vi "Config Info Get.vi"(8 "错误输入":errorcluster, 11 "Config Info":T8) -> (0 "错误输出":errorcluster, 1 "PLC Comms":T1={"PLC boolean read Tags"={"AT glass position"={"Tag Name"="S060.PXI.Signals.PlltData.SN", "Network Path"="172.15.51.1,1,0", "use opc"=FALSE, "DataSocket Reference"={"CWDSLib._DCWDataSocket"=refnum, "CWDSLib._DCWData"=refnum, "OnDataUpdated"=0, "OnStatusUpdated"=0}}, "AT shade position"={"Tag Name"="S060.PXI.Signals.PlltData.SN", "Network Path"="172.15.51.1,1,0", "use opc"=FALSE, "DataSocket Reference"={"CWDSLib._DCWDataSocket"=refnum, "CWDSLib._DCWData"=refnum, "OnDataUpdated"=0, "OnStatusUpdated"=0}}, "AT in glass wand lower pos"={"Tag Name"="S060.PXI.Signals.PlltData.SN", "Network Path"="172.15.51.1,1,0", "use opc"=FALSE, "DataSocket Reference"={"CWDSLib._DCWDataSocket"=refnum, "CWDSLib._DCWData"=refnum, "OnDataUpdated"=0, "OnStatusUpdated"=0}}, "AT in glass wand up pos"={"Tag Name"="S060.PXI.Signals.PlltData.SN", "Network Path"="172.15.51.1,1,0", "use opc"=FALSE, "DataSocket Reference"={"CWDSLib._DCWDataSocket"=refnum, "CWDSLib._DCWData"=refnum, "OnDataUpdated"=0, "OnStatusUpdated"=0}}, "AT in sunshad wand lower pos"={"Tag Name"="S060.PXI.Signals.PlltData.SN", "Network Path"="172.15.51.1,1,0", "use opc"=FALSE, "DataSocket Reference"={"CWDSLib._DCWDataSocket"=refnum, "CWDSLib._DCWData"=refnum, "OnDataUpdated"=0, "OnStatusUpdated"=0}}, "AT in sunshad wand up pos"={"Tag Name"="S060.PXI.Signals.PlltData.SN", "Network Path"="172.15.51.1,1,0", "use opc"=FALSE, "DataSocket Reference"={"CWDSLib._DCWDataSocket"=refnum, "CWDSLib._DCWData"=refnum, "OnDataUpdated"=0, "OnStatusUpdated"=0}}, "AT in wand home pos"={"Tag Name"="S060.PXI.Signals.PlltData.SN", "Network Path"="172.15.51.1,1,0", "use opc"=FALSE, "DataSocket Reference"={"CWDSLib._DCWDataSocket"=refnum, "CWDSLib._DCWData"=refnum, "OnDataUpdated"=0, "OnStatusUpdated"=0}}, "LVDT's Extended"={"Tag Name"="S060.PXI.Signals.PlltData.SN", "Network Path"="172.15.51.1,1,0", "use opc"=FALSE, "DataSocket Reference"={"CWDSLib._DCWDataSocket"=refnum, "CWDSLib._DCWData"=refnum, "OnDataUpdated"=0, "OnStatusUpdated"=0}}, "bolt check 1"={"Tag Name"="S060.PXI.Signals.PlltData.SN", "Network Path"="172.15.51.1,1,0", "use opc"=FALSE, "DataSocket Reference"={"CWDSLib._DCWDataSocket"=refnum, "CWDSLib._DCWData"=refnum, "OnDataUpdated"=0, "OnStatusUpdated"=0}}, "bolt check 2"={"Tag Name"="S060.PXI.Signals.PlltData.SN", "Network Path"="172.15.51.1,1,0", "use opc"=FALSE, "DataSocket Reference"={"CWDSLib._DCWDataSocket"=refnum, "CWDSLib._DCWData"=refnum, "OnDataUpdated"=0, "OnStatusUpdated"=0}}, "bolt check 3"={"Tag Name"="S060.PXI.Signals.PlltData.SN", "Network Path"="172.15.51.1,1,0", "use opc"=FALSE, "DataSocket Reference"={"CWDSLib._DCWDataSocket"=refnum, "CWDSLib._DCWData"=refnum, "OnDataUpdated"=0, "OnStatusUpdated"=0}}, "bolt check 4"={"Tag Name"="S060.PXI.Signals.PlltData.SN", "Network Path"="172.15.51.1,1,0", "use opc"=FALSE, "DataSocket Reference"={"CWDSLib._DCWDataSocket"=refnum, "CWDSLib._DCWData"=refnum, "OnDataUpdated"=0, "OnStatusUpdated"=0}}, "bolt check 5"={"Tag Name"="S060.PXI.Signals.PlltData.SN", "Network Path"="172.15.51.1,1,0", "use opc"=FALSE, "DataSocket Reference"={"CWDSLib._DCWDataSocket"=refnum, "CWDSLib._DCWData"=refnum, "OnDataUpdated"=0, "OnStatusUpdated"=0}}, "bolt check 6"={"Tag Name"="S060.PXI.Signals.PlltData.SN", "Network Path"="172.15.51.1,1,0", "use opc"=FALSE, "DataSocket Reference"={"CWDSLib._DCWDataSocket"=refnum, "CWDSLib._DCWData"=refnum, "OnDataUpdated"=0, "OnStatusUpdated"=0}}, "bolt check 7"={"Tag Name"="S060.PXI.Signals.PlltData.SN", "Network Path"="172.15.51.1,1,0", "use opc"=FALSE, "DataSocket Reference"={"CWDSLib._DCWDataSocket"=refnum, "CWDSLib._DCWData"=refnum, "OnDataUpdated"=0, "OnStatusUpdated"=0}}, "bolt check 8"={"Tag Name"="S060.PXI.Signals.PlltData.SN", "Network Path"="172.15.51.1,1,0", "use opc"=FALSE, "DataSocket Reference"={"CWDSLib._DCWDataSocket"=refnum, "CWDSLib._DCWData"=refnum, "OnDataUpdated"=0, "OnStatusUpdated"=0}}, "start"={"Tag Name"="S060.PXI.Signals.PlltData.SN", "Network Path"="172.15.51.1,1,0", "use opc"=FALSE, "DataSocket Reference"={"CWDSLib._DCWDataSocket"=refnum, "CWDSLib._DCWData"=refnum, "OnDataUpdated"=0, "OnStatusUpdated"=0}}, "abort"={"Tag Name"="S060.PXI.Signals.PlltData.SN", "Network Path"="172.15.51.1,1,0", "use opc"=FALSE, "DataSocket Reference"={"CWDSLib._DCWDataSocket"=refnum, "CWDSLib._DCWData"=refnum, "OnDataUpdated"=0, "OnStatusUpdated"=0}}, "LVDT's Retracted"={"Tag Name"="S060.PXI.Signals.PlltData.SN", "Network Path"="172.15.51.1,1,0", "use opc"=FALSE, "DataSocket Reference"={"CWDSLib._DCWDataSocket"=refnum, "CWDSLib._DCWData"=refnum, "OnDataUpdated"=0, "OnStatusUpdated"=0}}, "manual barcode print"={"Tag Name"="S060.PXI.Signals.PlltData.SN", "Network Path"="172.15.51.1,1,0", "use opc"=FALSE, "DataSocket Reference"={"CWDSLib._DCWDataSocket"=refnum, "CWDSLib._DCWData"=refnum, "OnDataUpdated"=0, "OnStatusUpdated"=0}}, "ss servo at open"={"Tag Name"="S060.PXI.Signals.PlltData.SN", "Network Path"="172.15.51.1,1,0", "use opc"=FALSE, "DataSocket Reference"={"CWDSLib._DCWDataSocket"=refnum, "CWDSLib._DCWData"=refnum, "OnDataUpdated"=0, "OnStatusUpdated"=0}}, "ss servo at close"={"Tag Name"="S060.PXI.Signals.PlltData.SN", "Network Path"="172.15.51.1,1,0", "use opc"=FALSE, "DataSocket Reference"={"CWDSLib._DCWDataSocket"=refnum, "CWDSLib._DCWData"=refnum, "OnDataUpdated"=0, "OnStatusUpdated"=0}}, "ss servo opening"={"Tag Name"="S060.PXI.Signals.PlltData.SN", "Network Path"="172.15.51.1,1,0", "use opc"=FALSE, "DataSocket Reference"={"CWDSLib._DCWDataSocket"=refnum, "CWDSLib._DCWData"=refnum, "OnDataUpdated"=0, "OnStatusUpdated"=0}}, "ss servo closing"={"Tag Name"="S060.PXI.Signals.PlltData.SN", "Network Path"="172.15.51.1,1,0", "use opc"=FALSE, "DataSocket Reference"={"CWDSLib._DCWDataSocket"=refnum, "CWDSLib._DCWData"=refnum, "OnDataUpdated"=0, "OnStatusUpdated"=0}}, "control slide at home"={"Tag Name"="S060.PXI.Signals.PlltData.SN", "Network Path"="172.15.51.1,1,0", "use opc"=FALSE, "DataSocket Reference"={"CWDSLib._DCWDataSocket"=refnum, "CWDSLib._DCWData"=refnum, "OnDataUpdated"=0, "OnStatusUpdated"=0}}, "control slide left good"={"Tag Name"="S060.PXI.Signals.PlltData.SN", "Network Path"="172.15.51.1,1,0", "use opc"=FALSE, "DataSocket Reference"={"CWDSLib._DCWDataSocket"=refnum, "CWDSLib._DCWData"=refnum, "OnDataUpdated"=0, "OnStatusUpdated"=0}}, "control slide left over stroke"={"Tag Name"="S060.PXI.Signals.PlltData.SN", "Network Path"="172.15.51.1,1,0", "use opc"=FALSE, "DataSocket Reference"={"CWDSLib._DCWDataSocket"=refnum, "CWDSLib._DCWData"=refnum, "OnDataUpdated"=0, "OnStatusUpdated"=0}}, "control slide right good"={"Tag Name"="S060.PXI.Signals.PlltData.SN", "Network Path"="172.15.51.1,1,0", "use opc"=FALSE, "DataSocket Reference"={"CWDSLib._DCWDataSocket"=refnum, "CWDSLib._DCWData"=refnum, "OnDataUpdated"=0, "OnStatusUpdated"=0}}, "control slide right over stroke"={"Tag Name"="S060.PXI.Signals.PlltData.SN", "Network Path"="172.15.51.1,1,0", "use opc"=FALSE, "DataSocket Reference"={"CWDSLib._DCWDataSocket"=refnum, "CWDSLib._DCWData"=refnum, "OnDataUpdated"=0, "OnStatusUpdated"=0}}, "wind deflector high speed pos"={"Tag Name"="S060.PXI.Signals.PlltData.SN", "Network Path"="172.15.51.1,1,0", "use opc"=FALSE, "DataSocket Reference"={"CWDSLib._DCWDataSocket"=refnum, "CWDSLib._DCWData"=refnum, "OnDataUpdated"=0, "OnStatusUpdated"=0}}, "wind deflector low speed pos"={"Tag Name"="S060.PXI.Signals.PlltData.SN", "Network Path"="172.15.51.1,1,0", "use opc"=FALSE, "DataSocket Reference"={"CWDSLib._DCWDataSocket"=refnum, "CWDSLib._DCWData"=refnum, "OnDataUpdated"=0, "OnStatusUpdated"=0}}, "AT VentPMACatHome"={"Tag Name"="S060.PXI.Signals.PlltData.SN", "Network Path"="172.15.51.1,1,0", "use opc"=FALSE, "DataSocket Reference"={"CWDSLib._DCWDataSocket"=refnum, "CWDSLib._DCWData"=refnum, "OnDataUpdated"=0, "OnStatusUpdated"=0}}, "AT VentPMACisExtend"={"Tag Name"="S060.PXI.Signals.PlltData.SN", "Network Path"="172.15.51.1,1,0", "use opc"=FALSE, "DataSocket Reference"={"CWDSLib._DCWDataSocket"=refnum, "CWDSLib._DCWData"=refnum, "OnDataUpdated"=0, "OnStatusUpdated"=0}}, "SS Barcode Scanner Bypassed"={"Tag Name"="S060.PXI.Signals.PlltData.SN", "Network Path"="172.15.51.1,1,0", "use opc"=FALSE, "DataSocket Reference"={"CWDSLib._DCWDataSocket"=refnum, "CWDSLib._DCWData"=refnum, "OnDataUpdated"=0, "OnStatusUpdated"=0}}, "Check Frame Barcode"={"Tag Name"="S060.PXI.Signals.PlltData.SN", "Network Path"="172.15.51.1,1,0", "use opc"=FALSE, "DataSocket Reference"={"CWDSLib._DCWDataSocket"=refnum, "CWDSLib._DCWData"=refnum, "OnDataUpdated"=0, "OnStatusUpdated"=0}}, "Z LVDTs Extended"={"Tag Name"="S060.PXI.Signals.PlltData.SN", "Network Path"="172.15.51.1,1,0", "use opc"=FALSE, "DataSocket Reference"={"CWDSLib._DCWDataSocket"=refnum, "CWDSLib._DCWData"=refnum, "OnDataUpdated"=0, "OnStatusUpdated"=0}}, "NVH Operator Pass"={"Tag Name"="S060.PXI.Signals.PlltData.SN", "Network Path"="172.15.51.1,1,0", "use opc"=FALSE, "DataSocket Reference"={"CWDSLib._DCWDataSocket"=refnum, "CWDSLib._DCWData"=refnum, "OnDataUpdated"=0, "OnStatusUpdated"=0}}, "NVH Operator Fail"={"Tag Name"="S060.PXI.Signals.PlltData.SN", "Network Path"="172.15.51.1,1,0", "use opc"=FALSE, "DataSocket Reference"={"CWDSLib._DCWDataSocket"=refnum, "CWDSLib._DCWData"=refnum, "OnDataUpdated"=0, "OnStatusUpdated"=0}}, "NVH Operator Express Glass Open"={"Tag Name"="S060.PXI.Signals.PlltData.SN", "Network Path"="172.15.51.1,1,0", "use opc"=FALSE, "DataSocket Reference"={"CWDSLib._DCWDataSocket"=refnum, "CWDSLib._DCWData"=refnum, "OnDataUpdated"=0, "OnStatusUpdated"=0}}, "NVH Operator Express Glass Close"={"Tag Name"="S060.PXI.Signals.PlltData.SN", "Network Path"="172.15.51.1,1,0", "use opc"=FALSE, "DataSocket Reference"={"CWDSLib._DCWDataSocket"=refnum, "CWDSLib._DCWData"=refnum, "OnDataUpdated"=0, "OnStatusUpdated"=0}}, "NVH Operator Express Rollo Open01"={"Tag Name"="S060.PXI.Signals.PlltData.SN", "Network Path"="172.15.51.1,1,0", "use opc"=FALSE, "DataSocket Reference"={"CWDSLib._DCWDataSocket"=refnum, "CWDSLib._DCWData"=refnum, "OnDataUpdated"=0, "OnStatusUpdated"=0}}, "NVH Operator Express Rollo Close01"={"Tag Name"="S060.PXI.Signals.PlltData.SN", "Network Path"="172.15.51.1,1,0", "use opc"=FALSE, "DataSocket Reference"={"CWDSLib._DCWDataSocket"=refnum, "CWDSLib._DCWData"=refnum, "OnDataUpdated"=0, "OnStatusUpdated"=0}}, "NVH Operator Express Rollo Open02"={"Tag Name"="S060.PXI.Signals.PlltData.SN", "Network Path"="172.15.51.1,1,0", "use opc"=FALSE, "DataSocket Reference"={"CWDSLib._DCWDataSocket"=refnum, "CWDSLib._DCWData"=refnum, "OnDataUpdated"=0, "OnStatusUpdated"=0}}, "NVH Operator Express Rollo Close02"={"Tag Name"="S060.PXI.Signals.PlltData.SN", "Network Path"="172.15.51.1,1,0", "use opc"=FALSE, "DataSocket Reference"={"CWDSLib._DCWDataSocket"=refnum, "CWDSLib._DCWData"=refnum, "OnDataUpdated"=0, "OnStatusUpdated"=0}}, "NVH Operator Vent Open Noise"={"Tag Name"="S060.PXI.Signals.PlltData.SN", "Network Path"="172.15.51.1,1,0", "use opc"=FALSE, "DataSocket Reference"={"CWDSLib._DCWDataSocket"=refnum, "CWDSLib._DCWData"=refnum, "OnDataUpdated"=0, "OnStatusUpdated"=0}}, "NVH Operator Vent Close Noise"={"Tag Name"="S060.PXI.Signals.PlltData.SN", "Network Path"="172.15.51.1,1,0", "use opc"=FALSE, "DataSocket Reference"={"CWDSLib._DCWDataSocket"=refnum, "CWDSLib._DCWData"=refnum, "OnDataUpdated"=0, "OnStatusUpdated"=0}}, "NVH Operator Sunshade Open Noise"={"Tag Name"="S060.PXI.Signals.PlltData.SN", "Network Path"="172.15.51.1,1,0", "use opc"=FALSE, "DataSocket Reference"={"CWDSLib._DCWDataSocket"=refnum, "CWDSLib._DCWData"=refnum, "OnDataUpdated"=0, "OnStatusUpdated"=0}}, "NVH Operator Sunshade Close Noise"={"Tag Name"="S060.PXI.Signals.PlltData.SN", "Network Path"="172.15.51.1,1,0", "use opc"=FALSE, "DataSocket Reference"={"CWDSLib._DCWDataSocket"=refnum, "CWDSLib._DCWData"=refnum, "OnDataUpdated"=0, "OnStatusUpdated"=0}}, "NVH Operator Glass Open Noise"={"Tag Name"="S060.PXI.Signals.PlltData.SN", "Network Path"="172.15.51.1,1,0", "use opc"=FALSE, "DataSocket Reference"={"CWDSLib._DCWDataSocket"=refnum, "CWDSLib._DCWData"=refnum, "OnDataUpdated"=0, "OnStatusUpdated"=0}}, "NVH Operator Glass Close Noise"={"Tag Name"="S060.PXI.Signals.PlltData.SN", "Network Path"="172.15.51.1,1,0", "use opc"=FALSE, "DataSocket Reference"={"CWDSLib._DCWDataSocket"=refnum, "CWDSLib._DCWData"=refnum, "OnDataUpdated"=0, "OnStatusUpdated"=0}}, "NVH Operator Finish"={"Tag Name"="S060.PXI.Signals.PlltData.SN", "Network Path"="172.15.51.1,1,0", "use opc"=FALSE, "DataSocket Reference"={"CWDSLib._DCWDataSocket"=refnum, "CWDSLib._DCWData"=refnum, "OnDataUpdated"=0, "OnStatusUpdated"=0}}, "NVH Operator Check"={"Tag Name"="S060.PXI.Signals.PlltData.SN", "Network Path"="172.15.51.1,1,0", "use opc"=FALSE, "DataSocket Reference"={"CWDSLib._DCWDataSocket"=refnum, "CWDSLib._DCWData"=refnum, "OnDataUpdated"=0, "OnStatusUpdated"=0}}, "windproof position"={"Tag Name"="S060.PXI.Signals.PlltData.SN", "Network Path"="172.15.51.1,1,0", "use opc"=FALSE, "DataSocket Reference"={"CWDSLib._DCWDataSocket"=refnum, "CWDSLib._DCWData"=refnum, "OnDataUpdated"=0, "OnStatusUpdated"=0}}, "NVH Operator Express Glass vent Open"={"Tag Name"="S060.PXI.Signals.PlltData.SN", "Network Path"="172.15.51.1,1,0", "use opc"=FALSE, "DataSocket Reference"={"CWDSLib._DCWDataSocket"=refnum, "CWDSLib._DCWData"=refnum, "OnDataUpdated"=0, "OnStatusUpdated"=0}}, "NVH Operator Express Glass Vent Close"={"Tag Name"="S060.PXI.Signals.PlltData.SN", "Network Path"="172.15.51.1,1,0", "use opc"=FALSE, "DataSocket Reference"={"CWDSLib._DCWDataSocket"=refnum, "CWDSLib._DCWData"=refnum, "OnDataUpdated"=0, "OnStatusUpdated"=0}}, "NVH Operator Re-do"={"Tag Name"="S060.PXI.Signals.PlltData.SN", "Network Path"="172.15.51.1,1,0", "use opc"=FALSE, "DataSocket Reference"={"CWDSLib._DCWDataSocket"=refnum, "CWDSLib._DCWData"=refnum, "OnDataUpdated"=0, "OnStatusUpdated"=0}}, "AT at vent ATS test pos"={"Tag Name"="S060.PXI.Signals.PlltData.SN", "Network Path"="172.15.51.1,1,0", "use opc"=FALSE, "DataSocket Reference"={"CWDSLib._DCWDataSocket"=refnum, "CWDSLib._DCWData"=refnum, "OnDataUpdated"=0, "OnStatusUpdated"=0}}, "AT at vent ATS Home pos"={"Tag Name"="S060.PXI.Signals.PlltData.SN", "Network Path"="172.15.51.1,1,0", "use opc"=FALSE, "DataSocket Reference"={"CWDSLib._DCWDataSocket"=refnum, "CWDSLib._DCWData"=refnum, "OnDataUpdated"=0, "OnStatusUpdated"=0}}, "Start Adjust LVDT"={"Tag Name"="S060.PXI.Signals.PlltData.SN", "Network Path"="172.15.51.1,1,0", "use opc"=FALSE, "DataSocket Reference"={"CWDSLib._DCWDataSocket"=refnum, "CWDSLib._DCWData"=refnum, "OnDataUpdated"=0, "OnStatusUpdated"=0}}, "Finish Adjust LVDT"={"Tag Name"="S060.PXI.Signals.PlltData.SN", "Network Path"="172.15.51.1,1,0", "use opc"=FALSE, "DataSocket Reference"={"CWDSLib._DCWDataSocket"=refnum, "CWDSLib._DCWData"=refnum, "OnDataUpdated"=0, "OnStatusUpdated"=0}}}, "PLC bool write Tags"={"AT set glass wand lower"={"Tag Name"="S060.PXI.Signals.PlltData.SN", "Network Path"="172.15.51.1,1,0", "use opc"=FALSE, "DataSocket Reference"={"CWDSLib._DCWDataSocket"=refnum, "CWDSLib._DCWData"=refnum, "OnDataUpdated"=0, "OnStatusUpdated"=0}}, "AT set sunshade wand lower"={"Tag Name"="S060.PXI.Signals.PlltData.SN", "Network Path"="172.15.51.1,1,0", "use opc"=FALSE, "DataSocket Reference"={"CWDSLib._DCWDataSocket"=refnum, "CWDSLib._DCWData"=refnum, "OnDataUpdated"=0, "OnStatusUpdated"=0}}, "AT set sunshade wand up"={"Tag Name"="S060.PXI.Signals.PlltData.SN", "Network Path"="172.15.51.1,1,0", "use opc"=FALSE, "DataSocket Reference"={"CWDSLib._DCWDataSocket"=refnum, "CWDSLib._DCWData"=refnum, "OnDataUpdated"=0, "OnStatusUpdated"=0}}, "AT set glass wand up"={"Tag Name"="S060.PXI.Signals.PlltData.SN", "Network Path"="172.15.51.1,1,0", "use opc"=FALSE, "DataSocket Reference"={"CWDSLib._DCWDataSocket"=refnum, "CWDSLib._DCWData"=refnum, "OnDataUpdated"=0, "OnStatusUpdated"=0}}, "AT set wand home pos"={"Tag Name"="S060.PXI.Signals.PlltData.SN", "Network Path"="172.15.51.1,1,0", "use opc"=FALSE, "DataSocket Reference"={"CWDSLib._DCWDataSocket"=refnum, "CWDSLib._DCWData"=refnum, "OnDataUpdated"=0, "OnStatusUpdated"=0}}, "Test Complete Pass"={"Tag Name"="S060.PXI.Signals.PlltData.SN", "Network Path"="172.15.51.1,1,0", "use opc"=FALSE, "DataSocket Reference"={"CWDSLib._DCWDataSocket"=refnum, "CWDSLib._DCWData"=refnum, "OnDataUpdated"=0, "OnStatusUpdated"=0}}, "Test Complete Fail"={"Tag Name"="S060.PXI.Signals.PlltData.SN", "Network Path"="172.15.51.1,1,0", "use opc"=FALSE, "DataSocket Reference"={"CWDSLib._DCWDataSocket"=refnum, "CWDSLib._DCWData"=refnum, "OnDataUpdated"=0, "OnStatusUpdated"=0}}, "Test Started"={"Tag Name"="S060.PXI.Signals.PlltData.SN", "Network Path"="172.15.51.1,1,0", "use opc"=FALSE, "DataSocket Reference"={"CWDSLib._DCWDataSocket"=refnum, "CWDSLib._DCWData"=refnum, "OnDataUpdated"=0, "OnStatusUpdated"=0}}, "Retract LVDT's"={"Tag Name"="S060.PXI.Signals.PlltData.SN", "Network Path"="172.15.51.1,1,0", "use opc"=FALSE, "DataSocket Reference"={"CWDSLib._DCWDataSocket"=refnum, "CWDSLib._DCWData"=refnum, "OnDataUpdated"=0, "OnStatusUpdated"=0}}, "Extend LVDT's"={"Tag Name"="S060.PXI.Signals.PlltData.SN", "Network Path"="172.15.51.1,1,0", "use opc"=FALSE, "DataSocket Reference"={"CWDSLib._DCWDataSocket"=refnum, "CWDSLib._DCWData"=refnum, "OnDataUpdated"=0, "OnStatusUpdated"=0}}, "ss servo open"={"Tag Name"="S060.PXI.Signals.PlltData.SN", "Network Path"="172.15.51.1,1,0", "use opc"=FALSE, "DataSocket Reference"={"CWDSLib._DCWDataSocket"=refnum, "CWDSLib._DCWData"=refnum, "OnDataUpdated"=0, "OnStatusUpdated"=0}}, "ss servo close"={"Tag Name"="S060.PXI.Signals.PlltData.SN", "Network Path"="172.15.51.1,1,0", "use opc"=FALSE, "DataSocket Reference"={"CWDSLib._DCWDataSocket"=refnum, "CWDSLib._DCWData"=refnum, "OnDataUpdated"=0, "OnStatusUpdated"=0}}, "control slide start"={"Tag Name"="S060.PXI.Signals.PlltData.SN", "Network Path"="172.15.51.1,1,0", "use opc"=FALSE, "DataSocket Reference"={"CWDSLib._DCWDataSocket"=refnum, "CWDSLib._DCWData"=refnum, "OnDataUpdated"=0, "OnStatusUpdated"=0}}, "control slide stop"={"Tag Name"="S060.PXI.Signals.PlltData.SN", "Network Path"="172.15.51.1,1,0", "use opc"=FALSE, "DataSocket Reference"={"CWDSLib._DCWDataSocket"=refnum, "CWDSLib._DCWData"=refnum, "OnDataUpdated"=0, "OnStatusUpdated"=0}}, "AT VentPMACHome"={"Tag Name"="S060.PXI.Signals.PlltData.SN", "Network Path"="172.15.51.1,1,0", "use opc"=FALSE, "DataSocket Reference"={"CWDSLib._DCWDataSocket"=refnum, "CWDSLib._DCWData"=refnum, "OnDataUpdated"=0, "OnStatusUpdated"=0}}, "AT VentPMACExtended"={"Tag Name"="S060.PXI.Signals.PlltData.SN", "Network Path"="172.15.51.1,1,0", "use opc"=FALSE, "DataSocket Reference"={"CWDSLib._DCWDataSocket"=refnum, "CWDSLib._DCWData"=refnum, "OnDataUpdated"=0, "OnStatusUpdated"=0}}, "Good Frame Barcode"={"Tag Name"="S060.PXI.Signals.PlltData.SN", "Network Path"="172.15.51.1,1,0", "use opc"=FALSE, "DataSocket Reference"={"CWDSLib._DCWDataSocket"=refnum, "CWDSLib._DCWData"=refnum, "OnDataUpdated"=0, "OnStatusUpdated"=0}}, "Bad Frame Barcode"={"Tag Name"="S060.PXI.Signals.PlltData.SN", "Network Path"="172.15.51.1,1,0", "use opc"=FALSE, "DataSocket Reference"={"CWDSLib._DCWDataSocket"=refnum, "CWDSLib._DCWData"=refnum, "OnDataUpdated"=0, "OnStatusUpdated"=0}}, "Extend Z LVDTS"={"Tag Name"="S060.PXI.Signals.PlltData.SN", "Network Path"="172.15.51.1,1,0", "use opc"=FALSE, "DataSocket Reference"={"CWDSLib._DCWDataSocket"=refnum, "CWDSLib._DCWData"=refnum, "OnDataUpdated"=0, "OnStatusUpdated"=0}}, "NVH SunRoof Moving"={"Tag Name"="S060.PXI.Signals.PlltData.SN", "Network Path"="172.15.51.1,1,0", "use opc"=FALSE, "DataSocket Reference"={"CWDSLib._DCWDataSocket"=refnum, "CWDSLib._DCWData"=refnum, "OnDataUpdated"=0, "OnStatusUpdated"=0}}, "NVH SunRoof Stop"={"Tag Name"="S060.PXI.Signals.PlltData.SN", "Network Path"="172.15.51.1,1,0", "use opc"=FALSE, "DataSocket Reference"={"CWDSLib._DCWDataSocket"=refnum, "CWDSLib._DCWData"=refnum, "OnDataUpdated"=0, "OnStatusUpdated"=0}}, "NVH Pass"={"Tag Name"="S060.PXI.Signals.PlltData.SN", "Network Path"="172.15.51.1,1,0", "use opc"=FALSE, "DataSocket Reference"={"CWDSLib._DCWDataSocket"=refnum, "CWDSLib._DCWData"=refnum, "OnDataUpdated"=0, "OnStatusUpdated"=0}}, "NVH Fail"={"Tag Name"="S060.PXI.Signals.PlltData.SN", "Network Path"="172.15.51.1,1,0", "use opc"=FALSE, "DataSocket Reference"={"CWDSLib._DCWDataSocket"=refnum, "CWDSLib._DCWData"=refnum, "OnDataUpdated"=0, "OnStatusUpdated"=0}}, "NVH Operator Express Glass Opened"={"Tag Name"="S060.PXI.Signals.PlltData.SN", "Network Path"="172.15.51.1,1,0", "use opc"=FALSE, "DataSocket Reference"={"CWDSLib._DCWDataSocket"=refnum, "CWDSLib._DCWData"=refnum, "OnDataUpdated"=0, "OnStatusUpdated"=0}}, "NVH Operator Express Glass Closed"={"Tag Name"="S060.PXI.Signals.PlltData.SN", "Network Path"="172.15.51.1,1,0", "use opc"=FALSE, "DataSocket Reference"={"CWDSLib._DCWDataSocket"=refnum, "CWDSLib._DCWData"=refnum, "OnDataUpdated"=0, "OnStatusUpdated"=0}}, "NVH Operator Express Rollo Opened01"={"Tag Name"="S060.PXI.Signals.PlltData.SN", "Network Path"="172.15.51.1,1,0", "use opc"=FALSE, "DataSocket Reference"={"CWDSLib._DCWDataSocket"=refnum, "CWDSLib._DCWData"=refnum, "OnDataUpdated"=0, "OnStatusUpdated"=0}}, "NVH Operator Express Rollo Closed01"={"Tag Name"="S060.PXI.Signals.PlltData.SN", "Network Path"="172.15.51.1,1,0", "use opc"=FALSE, "DataSocket Reference"={"CWDSLib._DCWDataSocket"=refnum, "CWDSLib._DCWData"=refnum, "OnDataUpdated"=0, "OnStatusUpdated"=0}}, "NVH Operator Express Rollo Opened02"={"Tag Name"="S060.PXI.Signals.PlltData.SN", "Network Path"="172.15.51.1,1,0", "use opc"=FALSE, "DataSocket Reference"={"CWDSLib._DCWDataSocket"=refnum, "CWDSLib._DCWData"=refnum, "OnDataUpdated"=0, "OnStatusUpdated"=0}}, "NVH Operator Pass"={"Tag Name"="S060.PXI.Signals.PlltData.SN", "Network Path"="172.15.51.1,1,0", "use opc"=FALSE, "DataSocket Reference"={"CWDSLib._DCWDataSocket"=refnum, "CWDSLib._DCWData"=refnum, "OnDataUpdated"=0, "OnStatusUpdated"=0}}, "NVH Operator Fail"={"Tag Name"="S060.PXI.Signals.PlltData.SN", "Network Path"="172.15.51.1,1,0", "use opc"=FALSE, "DataSocket Reference"={"CWDSLib._DCWDataSocket"=refnum, "CWDSLib._DCWData"=refnum, "OnDataUpdated"=0, "OnStatusUpdated"=0}}, "NVH Operator Check"={"Tag Name"="S060.PXI.Signals.PlltData.SN", "Network Path"="172.15.51.1,1,0", "use opc"=FALSE, "DataSocket Reference"={"CWDSLib._DCWDataSocket"=refnum, "CWDSLib._DCWData"=refnum, "OnDataUpdated"=0, "OnStatusUpdated"=0}}, "NVH Operator Vent Open Noise"={"Tag Name"="S060.PXI.Signals.PlltData.SN", "Network Path"="172.15.51.1,1,0", "use opc"=FALSE, "DataSocket Reference"={"CWDSLib._DCWDataSocket"=refnum, "CWDSLib._DCWData"=refnum, "OnDataUpdated"=0, "OnStatusUpdated"=0}}, "NVH Operator Vent Close Noise"={"Tag Name"="S060.PXI.Signals.PlltData.SN", "Network Path"="172.15.51.1,1,0", "use opc"=FALSE, "DataSocket Reference"={"CWDSLib._DCWDataSocket"=refnum, "CWDSLib._DCWData"=refnum, "OnDataUpdated"=0, "OnStatusUpdated"=0}}, "NVH Operator Sunshade Open Noise"={"Tag Name"="S060.PXI.Signals.PlltData.SN", "Network Path"="172.15.51.1,1,0", "use opc"=FALSE, "DataSocket Reference"={"CWDSLib._DCWDataSocket"=refnum, "CWDSLib._DCWData"=refnum, "OnDataUpdated"=0, "OnStatusUpdated"=0}}, "NVH Operator Sunshade Close Noise"={"Tag Name"="S060.PXI.Signals.PlltData.SN", "Network Path"="172.15.51.1,1,0", "use opc"=FALSE, "DataSocket Reference"={"CWDSLib._DCWDataSocket"=refnum, "CWDSLib._DCWData"=refnum, "OnDataUpdated"=0, "OnStatusUpdated"=0}}, "NVH Operator Glass Open Noise"={"Tag Name"="S060.PXI.Signals.PlltData.SN", "Network Path"="172.15.51.1,1,0", "use opc"=FALSE, "DataSocket Reference"={"CWDSLib._DCWDataSocket"=refnum, "CWDSLib._DCWData"=refnum, "OnDataUpdated"=0, "OnStatusUpdated"=0}}, "NVH Operator Glass Close Noise"={"Tag Name"="S060.PXI.Signals.PlltData.SN", "Network Path"="172.15.51.1,1,0", "use opc"=FALSE, "DataSocket Reference"={"CWDSLib._DCWDataSocket"=refnum, "CWDSLib._DCWData"=refnum, "OnDataUpdated"=0, "OnStatusUpdated"=0}}, "NVH Operator Finish"={"Tag Name"="S060.PXI.Signals.PlltData.SN", "Network Path"="172.15.51.1,1,0", "use opc"=FALSE, "DataSocket Reference"={"CWDSLib._DCWDataSocket"=refnum, "CWDSLib._DCWData"=refnum, "OnDataUpdated"=0, "OnStatusUpdated"=0}}, "Barcode01 OK"={"Tag Name"="S060.PXI.Signals.PlltData.SN", "Network Path"="172.15.51.1,1,0", "use opc"=FALSE, "DataSocket Reference"={"CWDSLib._DCWDataSocket"=refnum, "CWDSLib._DCWData"=refnum, "OnDataUpdated"=0, "OnStatusUpdated"=0}}, "Barcode02 OK"={"Tag Name"="S060.PXI.Signals.PlltData.SN", "Network Path"="172.15.51.1,1,0", "use opc"=FALSE, "DataSocket Reference"={"CWDSLib._DCWDataSocket"=refnum, "CWDSLib._DCWData"=refnum, "OnDataUpdated"=0, "OnStatusUpdated"=0}}, "AT set to Vent ATS Test Pos"={"Tag Name"="S060.PXI.Signals.PlltData.SN", "Network Path"="172.15.51.1,1,0", "use opc"=FALSE, "DataSocket Reference"={"CWDSLib._DCWDataSocket"=refnum, "CWDSLib._DCWData"=refnum, "OnDataUpdated"=0, "OnStatusUpdated"=0}}, "AT set to Vent ATS Home Pos"={"Tag Name"="S060.PXI.Signals.PlltData.SN", "Network Path"="172.15.51.1,1,0", "use opc"=FALSE, "DataSocket Reference"={"CWDSLib._DCWDataSocket"=refnum, "CWDSLib._DCWData"=refnum, "OnDataUpdated"=0, "OnStatusUpdated"=0}}, "Move LVDT Adjust Station"={"Tag Name"="S060.PXI.Signals.PlltData.SN", "Network Path"="172.15.51.1,1,0", "use opc"=FALSE, "DataSocket Reference"={"CWDSLib._DCWDataSocket"=refnum, "CWDSLib._DCWData"=refnum, "OnDataUpdated"=0, "OnStatusUpdated"=0}}}, "PLC string read Tags"={"Serial Number"={"Tag Name"="S060.PXI.Signals.PlltData.SN", "Network Path"="172.15.51.1,1,0", "use opc"=FALSE, "DataSocket Reference"={"CWDSLib._DCWDataSocket"=refnum, "CWDSLib._DCWData"=refnum, "OnDataUpdated"=0, "OnStatusUpdated"=0}}, "Pallet Number"={"Tag Name"="S060.PXI.Signals.PlltData.SN", "Network Path"="172.15.51.1,1,0", "use opc"=FALSE, "DataSocket Reference"={"CWDSLib._DCWDataSocket"=refnum, "CWDSLib._DCWData"=refnum, "OnDataUpdated"=0, "OnStatusUpdated"=0}}, "Inalfa Part Number"={"Tag Name"="S060.PXI.Signals.PlltData.SN", "Network Path"="172.15.51.1,1,0", "use opc"=FALSE, "DataSocket Reference"={"CWDSLib._DCWDataSocket"=refnum, "CWDSLib._DCWData"=refnum, "OnDataUpdated"=0, "OnStatusUpdated"=0}}, "Shade Color"={"Tag Name"="S060.PXI.Signals.PlltData.SN", "Network Path"="172.15.51.1,1,0", "use opc"=FALSE, "DataSocket Reference"={"CWDSLib._DCWDataSocket"=refnum, "CWDSLib._DCWData"=refnum, "OnDataUpdated"=0, "OnStatusUpdated"=0}}, "Model Type"={"Tag Name"="S060.PXI.Signals.PlltData.SN", "Network Path"="172.15.51.1,1,0", "use opc"=FALSE, "DataSocket Reference"={"CWDSLib._DCWDataSocket"=refnum, "CWDSLib._DCWData"=refnum, "OnDataUpdated"=0, "OnStatusUpdated"=0}}, "Customer Number"={"Tag Name"="S060.PXI.Signals.PlltData.SN", "Network Path"="172.15.51.1,1,0", "use opc"=FALSE, "DataSocket Reference"={"CWDSLib._DCWDataSocket"=refnum, "CWDSLib._DCWData"=refnum, "OnDataUpdated"=0, "OnStatusUpdated"=0}}, "Part History Number"={"Tag Name"="S060.PXI.Signals.PlltData.SN", "Network Path"="172.15.51.1,1,0", "use opc"=FALSE, "DataSocket Reference"={"CWDSLib._DCWDataSocket"=refnum, "CWDSLib._DCWData"=refnum, "OnDataUpdated"=0, "OnStatusUpdated"=0}}, "Shade 1 Barcode"={"Tag Name"="S060.PXI.Signals.PlltData.SN", "Network Path"="172.15.51.1,1,0", "use opc"=FALSE, "DataSocket Reference"={"CWDSLib._DCWDataSocket"=refnum, "CWDSLib._DCWData"=refnum, "OnDataUpdated"=0, "OnStatusUpdated"=0}}, "Shade 2 Barcode"={"Tag Name"="S060.PXI.Signals.PlltData.SN", "Network Path"="172.15.51.1,1,0", "use opc"=FALSE, "DataSocket Reference"={"CWDSLib._DCWDataSocket"=refnum, "CWDSLib._DCWData"=refnum, "OnDataUpdated"=0, "OnStatusUpdated"=0}}, "Manual Serial Number"={"Tag Name"="S060.PXI.Signals.PlltData.SN", "Network Path"="172.15.51.1,1,0", "use opc"=FALSE, "DataSocket Reference"={"CWDSLib._DCWDataSocket"=refnum, "CWDSLib._DCWData"=refnum, "OnDataUpdated"=0, "OnStatusUpdated"=0}}, "Manual Inalfa Part Number"={"Tag Name"="S060.PXI.Signals.PlltData.SN", "Network Path"="172.15.51.1,1,0", "use opc"=FALSE, "DataSocket Reference"={"CWDSLib._DCWDataSocket"=refnum, "CWDSLib._DCWData"=refnum, "OnDataUpdated"=0, "OnStatusUpdated"=0}}, "Manual Shade Color"={"Tag Name"="S060.PXI.Signals.PlltData.SN", "Network Path"="172.15.51.1,1,0", "use opc"=FALSE, "DataSocket Reference"={"CWDSLib._DCWDataSocket"=refnum, "CWDSLib._DCWData"=refnum, "OnDataUpdated"=0, "OnStatusUpdated"=0}}, "Manual Model Type"={"Tag Name"="S060.PXI.Signals.PlltData.SN", "Network Path"="172.15.51.1,1,0", "use opc"=FALSE, "DataSocket Reference"={"CWDSLib._DCWDataSocket"=refnum, "CWDSLib._DCWData"=refnum, "OnDataUpdated"=0, "OnStatusUpdated"=0}}, "Manual Customer Number"={"Tag Name"="S060.PXI.Signals.PlltData.SN", "Network Path"="172.15.51.1,1,0", "use opc"=FALSE, "DataSocket Reference"={"CWDSLib._DCWDataSocket"=refnum, "CWDSLib._DCWData"=refnum, "OnDataUpdated"=0, "OnStatusUpdated"=0}}, "Manual Part History Number"={"Tag Name"="S060.PXI.Signals.PlltData.SN", "Network Path"="172.15.51.1,1,0", "use opc"=FALSE, "DataSocket Reference"={"CWDSLib._DCWDataSocket"=refnum, "CWDSLib._DCWData"=refnum, "OnDataUpdated"=0, "OnStatusUpdated"=0}}}, "PLC string write Tags"={"barcode station error"={"Tag Name"="S060.PXI.Signals.PlltData.SN", "Network Path"="172.15.51.1,1,0", "use opc"=FALSE, "DataSocket Reference"={"CWDSLib._DCWDataSocket"=refnum, "CWDSLib._DCWData"=refnum, "OnDataUpdated"=0, "OnStatusUpdated"=0}}, "error message 0"={"Tag Name"="S060.PXI.Signals.PlltData.SN", "Network Path"="172.15.51.1,1,0", "use opc"=FALSE, "DataSocket Reference"={"CWDSLib._DCWDataSocket"=refnum, "CWDSLib._DCWData"=refnum, "OnDataUpdated"=0, "OnStatusUpdated"=0}}, "error message 1"={"Tag Name"="S060.PXI.Signals.PlltData.SN", "Network Path"="172.15.51.1,1,0", "use opc"=FALSE, "DataSocket Reference"={"CWDSLib._DCWDataSocket"=refnum, "CWDSLib._DCWData"=refnum, "OnDataUpdated"=0, "OnStatusUpdated"=0}}, "error message 2"={"Tag Name"="S060.PXI.Signals.PlltData.SN", "Network Path"="172.15.51.1,1,0", "use opc"=FALSE, "DataSocket Reference"={"CWDSLib._DCWDataSocket"=refnum, "CWDSLib._DCWData"=refnum, "OnDataUpdated"=0, "OnStatusUpdated"=0}}, "error message 3"={"Tag Name"="S060.PXI.Signals.PlltData.SN", "Network Path"="172.15.51.1,1,0", "use opc"=FALSE, "DataSocket Reference"={"CWDSLib._DCWDataSocket"=refnum, "CWDSLib._DCWData"=refnum, "OnDataUpdated"=0, "OnStatusUpdated"=0}}}, "use opc"=FALSE, "PLC/OPC Path"=""} {"PLC string write Tags"."error message 3"."DataSocket Reference"."OnStatusUpdated" format="%.0x"; "PLC string write Tags"."error message 3"."DataSocket Reference"."OnDataUpdated" format="%.0x"; "PLC string write Tags"."error message 2"."DataSocket Reference"."OnStatusUpdated" format="%.0x"; "PLC string write Tags"."error message 2"."DataSocket Reference"."OnDataUpdated" format="%.0x"; "PLC string write Tags"."error message 1"."DataSocket Reference"."OnStatusUpdated" format="%.0x"; "PLC string write Tags"."error message 1"."DataSocket Reference"."OnDataUpdated" format="%.0x"; "PLC string write Tags"."error message 0"."DataSocket Reference"."OnStatusUpdated" format="%.0x"; "PLC string write Tags"."error message 0"."DataSocket Reference"."OnDataUpdated" format="%.0x"; "PLC string write Tags"."barcode station error"."DataSocket Reference"."OnStatusUpdated" format="%.0x"; "PLC string write Tags"."barcode station error"."DataSocket Reference"."OnDataUpdated" format="%.0x"; "PLC string read Tags"."Manual Part History Number"."DataSocket Reference"."OnStatusUpdated" format="%.0x"; "PLC string read Tags"."Manual Part History Number"."DataSocket Reference"."OnDataUpdated" format="%.0x"; "PLC string read Tags"."Manual Customer Number"."DataSocket Reference"."OnStatusUpdated" format="%.0x"; "PLC string read Tags"."Manual Customer Number"."DataSocket Reference"."OnDataUpdated" format="%.0x"; "PLC string read Tags"."Manual Model Type"."DataSocket Reference"."OnStatusUpdated" format="%.0x"; "PLC string read Tags"."Manual Model Type"."DataSocket Reference"."OnDataUpdated" format="%.0x"; "PLC string read Tags"."Manual Shade Color"."DataSocket Reference"."OnStatusUpdated" format="%.0x"; "PLC string read Tags"."Manual Shade Color"."DataSocket Reference"."OnDataUpdated" format="%.0x"; "PLC string read Tags"."Manual Inalfa Part Number"."DataSocket Reference"."OnStatusUpdated" format="%.0x"; "PLC string read Tags"."Manual Inalfa Part Number"."DataSocket Reference"."OnDataUpdated" format="%.0x"; "PLC string read Tags"."Manual Serial Number"."DataSocket Reference"."OnStatusUpdated" format="%.0x"; "PLC string read Tags"."Manual Serial Number"."DataSocket Reference"."OnDataUpdated" format="%.0x"; "PLC string read Tags"."Shade 2 Barcode"."DataSocket Reference"."OnStatusUpdated" format="%.0x"; "PLC string read Tags"."Shade 2 Barcode"."DataSocket Reference"."OnDataUpdated" format="%.0x"; "PLC string read Tags"."Shade 1 Barcode"."DataSocket Reference"."OnStatusUpdated" format="%.0x"; "PLC string read Tags"."Shade 1 Barcode"."DataSocket Reference"."OnDataUpdated" format="%.0x"; "PLC string read Tags"."Part History Number"."DataSocket Reference"."OnStatusUpdated" format="%.0x"; "PLC string read Tags"."Part History Number"."DataSocket Reference"."OnDataUpdated" format="%.0x"; "PLC string read Tags"."Customer Number"."DataSocket Reference"."OnStatusUpdated" format="%.0x"; "PLC string read Tags"."Customer Number"."DataSocket Reference"."OnDataUpdated" format="%.0x"; "PLC string read Tags"."Model Type"."DataSocket Reference"."OnStatusUpdated" format="%.0x"; "PLC string read Tags"."Model Type"."DataSocket Reference"."OnDataUpdated" format="%.0x"; "PLC string read Tags"."Shade Color"."DataSocket Reference"."OnStatusUpdated" format="%.0x"; "PLC string read Tags"."Shade Color"."DataSocket Reference"."OnDataUpdated" format="%.0x"; "PLC string read Tags"."Inalfa Part Number"."DataSocket Reference"."OnStatusUpdated" format="%.0x"; "PLC string read Tags"."Inalfa Part Number"."DataSocket Reference"."OnDataUpdated" format="%.0x"; "PLC string read Tags"."Pallet Number"."DataSocket Reference"."OnStatusUpdated" format="%.0x"; "PLC string read Tags"."Pallet Number"."DataSocket Reference"."OnDataUpdated" format="%.0x"; "PLC string read Tags"."Serial Number"."DataSocket Reference"."OnStatusUpdated" format="%.0x"; "PLC string read Tags"."Serial Number"."DataSocket Reference"."OnDataUpdated" format="%.0x"; "PLC bool write Tags"."Move LVDT Adjust Station"."DataSocket Reference"."OnStatusUpdated" format="%.0x"; "PLC bool write Tags"."Move LVDT Adjust Station"."DataSocket Reference"."OnDataUpdated" format="%.0x"; "PLC bool write Tags"."AT set to Vent ATS Home Pos"."DataSocket Reference"."OnStatusUpdated" format="%.0x"; "PLC bool write Tags"."AT set to Vent ATS Home Pos"."DataSocket Reference"."OnDataUpdated" format="%.0x"; "PLC bool write Tags"."AT set to Vent ATS Test Pos"."DataSocket Reference"."OnStatusUpdated" format="%.0x"; "PLC bool write Tags"."AT set to Vent ATS Test Pos"."DataSocket Reference"."OnDataUpdated" format="%.0x"; "PLC bool write Tags"."Barcode02 OK"."DataSocket Reference"."OnStatusUpdated" format="%.0x"; "PLC bool write Tags"."Barcode02 OK"."DataSocket Reference"."OnDataUpdated" format="%.0x"; "PLC bool write Tags"."Barcode01 OK"."DataSocket Reference"."OnStatusUpdated" format="%.0x"; "PLC bool write Tags"."Barcode01 OK"."DataSocket Reference"."OnDataUpdated" format="%.0x"; "PLC bool write Tags"."AT set glass wand up"."DataSocket Reference"."OnStatusUpdated" format="%.0x"; "PLC bool write Tags"."AT set glass wand up"."DataSocket Reference"."OnDataUpdated" format="%.0x"; "PLC bool write Tags"."AT set sunshade wand up"."DataSocket Reference"."OnStatusUpdated" format="%.0x"; "PLC bool write Tags"."AT set sunshade wand up"."DataSocket Reference"."OnDataUpdated" format="%.0x"; "PLC bool write Tags"."NVH Operator Finish"."DataSocket Reference"."OnStatusUpdated" format="%.0x"; "PLC bool write Tags"."NVH Operator Finish"."DataSocket Reference"."OnDataUpdated" format="%.0x"; "PLC bool write Tags"."NVH Operator Glass Close Noise"."DataSocket Reference"."OnStatusUpdated" format="%.0x"; "PLC bool write Tags"."NVH Operator Glass Close Noise"."DataSocket Reference"."OnDataUpdated" format="%.0x"; "PLC bool write Tags"."NVH Operator Glass Open Noise"."DataSocket Reference"."OnStatusUpdated" format="%.0x"; "PLC bool write Tags"."NVH Operator Glass Open Noise"."DataSocket Reference"."OnDataUpdated" format="%.0x"; "PLC bool write Tags"."NVH Operator Sunshade Close Noise"."DataSocket Reference"."OnStatusUpdated" format="%.0x"; "PLC bool write Tags"."NVH Operator Sunshade Close Noise"."DataSocket Reference"."OnDataUpdated" format="%.0x"; "PLC bool write Tags"."NVH Operator Sunshade Open Noise"."DataSocket Reference"."OnStatusUpdated" format="%.0x"; "PLC bool write Tags"."NVH Operator Sunshade Open Noise"."DataSocket Reference"."OnDataUpdated" format="%.0x"; "PLC bool write Tags"."NVH Operator Vent Close Noise"."DataSocket Reference"."OnStatusUpdated" format="%.0x"; "PLC bool write Tags"."NVH Operator Vent Close Noise"."DataSocket Reference"."OnDataUpdated" format="%.0x"; "PLC bool write Tags"."NVH Operator Vent Open Noise"."DataSocket Reference"."OnStatusUpdated" format="%.0x"; "PLC bool write Tags"."NVH Operator Vent Open Noise"."DataSocket Reference"."OnDataUpdated" format="%.0x"; "PLC bool write Tags"."NVH Operator Check"."DataSocket Reference"."OnStatusUpdated" format="%.0x"; "PLC bool write Tags"."NVH Operator Check"."DataSocket Reference"."OnDataUpdated" format="%.0x"; "PLC bool write Tags"."NVH Operator Fail"."DataSocket Reference"."OnStatusUpdated" format="%.0x"; "PLC bool write Tags"."NVH Operator Fail"."DataSocket Reference"."OnDataUpdated" format="%.0x"; "PLC bool write Tags"."NVH Operator Pass"."DataSocket Reference"."OnStatusUpdated" format="%.0x"; "PLC bool write Tags"."NVH Operator Pass"."DataSocket Reference"."OnDataUpdated" format="%.0x"; "PLC bool write Tags"."NVH Operator Express Rollo Opened02"."DataSocket Reference"."OnStatusUpdated" format="%.0x"; "PLC bool write Tags"."NVH Operator Express Rollo Opened02"."DataSocket Reference"."OnDataUpdated" format="%.0x"; "PLC bool write Tags"."NVH Operator Express Rollo Closed01"."DataSocket Reference"."OnStatusUpdated" format="%.0x"; "PLC bool write Tags"."NVH Operator Express Rollo Closed01"."DataSocket Reference"."OnDataUpdated" format="%.0x"; "PLC bool write Tags"."NVH Operator Express Rollo Opened01"."DataSocket Reference"."OnStatusUpdated" format="%.0x"; "PLC bool write Tags"."NVH Operator Express Rollo Opened01"."DataSocket Reference"."OnDataUpdated" format="%.0x"; "PLC bool write Tags"."NVH Operator Express Glass Closed"."DataSocket Reference"."OnStatusUpdated" format="%.0x"; "PLC bool write Tags"."NVH Operator Express Glass Closed"."DataSocket Reference"."OnDataUpdated" format="%.0x"; "PLC bool write Tags"."NVH Operator Express Glass Opened"."DataSocket Reference"."OnStatusUpdated" format="%.0x"; "PLC bool write Tags"."NVH Operator Express Glass Opened"."DataSocket Reference"."OnDataUpdated" format="%.0x"; "PLC bool write Tags"."NVH Fail"."DataSocket Reference"."OnStatusUpdated" format="%.0x"; "PLC bool write Tags"."NVH Fail"."DataSocket Reference"."OnDataUpdated" format="%.0x"; "PLC bool write Tags"."NVH Pass"."DataSocket Reference"."OnStatusUpdated" format="%.0x"; "PLC bool write Tags"."NVH Pass"."DataSocket Reference"."OnDataUpdated" format="%.0x"; "PLC bool write Tags"."NVH SunRoof Stop"."DataSocket Reference"."OnStatusUpdated" format="%.0x"; "PLC bool write Tags"."NVH SunRoof Stop"."DataSocket Reference"."OnDataUpdated" format="%.0x"; "PLC bool write Tags"."NVH SunRoof Moving"."DataSocket Reference"."OnStatusUpdated" format="%.0x"; "PLC bool write Tags"."NVH SunRoof Moving"."DataSocket Reference"."OnDataUpdated" format="%.0x"; "PLC bool write Tags"."Extend Z LVDTS"."DataSocket Reference"."OnStatusUpdated" format="%.0x"; "PLC bool write Tags"."Extend Z LVDTS"."DataSocket Reference"."OnDataUpdated" format="%.0x"; "PLC bool write Tags"."Bad Frame Barcode"."DataSocket Reference"."OnStatusUpdated" format="%.0x"; "PLC bool write Tags"."Bad Frame Barcode"."DataSocket Reference"."OnDataUpdated" format="%.0x"; "PLC bool write Tags"."Good Frame Barcode"."DataSocket Reference"."OnStatusUpdated" format="%.0x"; "PLC bool write Tags"."Good Frame Barcode"."DataSocket Reference"."OnDataUpdated" format="%.0x"; "PLC bool write Tags"."AT VentPMACExtended"."DataSocket Reference"."OnStatusUpdated" format="%.0x"; "PLC bool write Tags"."AT VentPMACExtended"."DataSocket Reference"."OnDataUpdated" format="%.0x"; "PLC bool write Tags"."AT VentPMACHome"."DataSocket Reference"."OnStatusUpdated" format="%.0x"; "PLC bool write Tags"."AT VentPMACHome"."DataSocket Reference"."OnDataUpdated" format="%.0x"; "PLC bool write Tags"."control slide stop"."DataSocket Reference"."OnStatusUpdated" format="%.0x"; "PLC bool write Tags"."control slide stop"."DataSocket Reference"."OnDataUpdated" format="%.0x"; "PLC bool write Tags"."control slide start"."DataSocket Reference"."OnStatusUpdated" format="%.0x"; "PLC bool write Tags"."control slide start"."DataSocket Reference"."OnDataUpdated" format="%.0x"; "PLC bool write Tags"."ss servo close"."DataSocket Reference"."OnStatusUpdated" format="%.0x"; "PLC bool write Tags"."ss servo close"."DataSocket Reference"."OnDataUpdated" format="%.0x"; "PLC bool write Tags"."ss servo open"."DataSocket Reference"."OnStatusUpdated" format="%.0x"; "PLC bool write Tags"."ss servo open"."DataSocket Reference"."OnDataUpdated" format="%.0x"; "PLC bool write Tags"."Extend LVDT's"."DataSocket Reference"."OnStatusUpdated" format="%.0x"; "PLC bool write Tags"."Extend LVDT's"."DataSocket Reference"."OnDataUpdated" format="%.0x"; "PLC bool write Tags"."Retract LVDT's"."DataSocket Reference"."OnStatusUpdated" format="%.0x"; "PLC bool write Tags"."Retract LVDT's"."DataSocket Reference"."OnDataUpdated" format="%.0x"; "PLC bool write Tags"."Test Started"."DataSocket Reference"."OnStatusUpdated" format="%.0x"; "PLC bool write Tags"."Test Started"."DataSocket Reference"."OnDataUpdated" format="%.0x"; "PLC bool write Tags"."Test Complete Fail"."DataSocket Reference"."OnStatusUpdated" format="%.0x"; "PLC bool write Tags"."Test Complete Fail"."DataSocket Reference"."OnDataUpdated" format="%.0x"; "PLC bool write Tags"."Test Complete Pass"."DataSocket Reference"."OnStatusUpdated" format="%.0x"; "PLC bool write Tags"."Test Complete Pass"."DataSocket Reference"."OnDataUpdated" format="%.0x"; "PLC bool write Tags"."AT set wand home pos"."DataSocket Reference"."OnStatusUpdated" format="%.0x"; "PLC bool write Tags"."AT set wand home pos"."DataSocket Reference"."OnDataUpdated" format="%.0x"; "PLC bool write Tags"."AT set sunshade wand lower"."DataSocket Reference"."OnStatusUpdated" format="%.0x"; "PLC bool write Tags"."AT set sunshade wand lower"."DataSocket Reference"."OnDataUpdated" format="%.0x"; "PLC bool write Tags"."AT set glass wand lower"."DataSocket Reference"."OnStatusUpdated" format="%.0x"; "PLC bool write Tags"."AT set glass wand lower"."DataSocket Reference"."OnDataUpdated" format="%.0x"; "PLC boolean read Tags"."AT in sunshad wand up pos"."DataSocket Reference"."OnStatusUpdated" format="%.0x"; "PLC boolean read Tags"."AT in sunshad wand up pos"."DataSocket Reference"."OnDataUpdated" format="%.0x"; "PLC boolean read Tags"."AT in glass wand up pos"."DataSocket Reference"."OnStatusUpdated" format="%.0x"; "PLC boolean read Tags"."AT in glass wand up pos"."DataSocket Reference"."OnDataUpdated" format="%.0x"; "PLC boolean read Tags"."Finish Adjust LVDT"."DataSocket Reference"."OnStatusUpdated" format="%.0x"; "PLC boolean read Tags"."Finish Adjust LVDT"."DataSocket Reference"."OnDataUpdated" format="%.0x"; "PLC boolean read Tags"."Start Adjust LVDT"."DataSocket Reference"."OnStatusUpdated" format="%.0x"; "PLC boolean read Tags"."Start Adjust LVDT"."DataSocket Reference"."OnDataUpdated" format="%.0x"; "PLC boolean read Tags"."AT at vent ATS Home pos"."DataSocket Reference"."OnStatusUpdated" format="%.0x"; "PLC boolean read Tags"."AT at vent ATS Home pos"."DataSocket Reference"."OnDataUpdated" format="%.0x"; "PLC boolean read Tags"."AT at vent ATS test pos"."DataSocket Reference"."OnStatusUpdated" format="%.0x"; "PLC boolean read Tags"."AT at vent ATS test pos"."DataSocket Reference"."OnDataUpdated" format="%.0x"; "PLC boolean read Tags"."NVH Operator Re-do"."DataSocket Reference"."OnStatusUpdated" format="%.0x"; "PLC boolean read Tags"."NVH Operator Re-do"."DataSocket Reference"."OnDataUpdated" format="%.0x"; "PLC boolean read Tags"."NVH Operator Express Glass Vent Close"."DataSocket Reference"."OnStatusUpdated" format="%.0x"; "PLC boolean read Tags"."NVH Operator Express Glass Vent Close"."DataSocket Reference"."OnDataUpdated" format="%.0x"; "PLC boolean read Tags"."NVH Operator Express Glass vent Open"."DataSocket Reference"."OnStatusUpdated" format="%.0x"; "PLC boolean read Tags"."NVH Operator Express Glass vent Open"."DataSocket Reference"."OnDataUpdated" format="%.0x"; "PLC boolean read Tags"."windproof position"."DataSocket Reference"."OnStatusUpdated" format="%.0x"; "PLC boolean read Tags"."windproof position"."DataSocket Reference"."OnDataUpdated" format="%.0x"; "PLC boolean read Tags"."NVH Operator Check"."DataSocket Reference"."OnStatusUpdated" format="%.0x"; "PLC boolean read Tags"."NVH Operator Check"."DataSocket Reference"."OnDataUpdated" format="%.0x"; "PLC boolean read Tags"."NVH Operator Finish"."DataSocket Reference"."OnStatusUpdated" format="%.0x"; "PLC boolean read Tags"."NVH Operator Finish"."DataSocket Reference"."OnDataUpdated" format="%.0x"; "PLC boolean read Tags"."NVH Operator Glass Close Noise"."DataSocket Reference"."OnStatusUpdated" format="%.0x"; "PLC boolean read Tags"."NVH Operator Glass Close Noise"."DataSocket Reference"."OnDataUpdated" format="%.0x"; "PLC boolean read Tags"."NVH Operator Glass Open Noise"."DataSocket Reference"."OnStatusUpdated" format="%.0x"; "PLC boolean read Tags"."NVH Operator Glass Open Noise"."DataSocket Reference"."OnDataUpdated" format="%.0x"; "PLC boolean read Tags"."NVH Operator Sunshade Close Noise"."DataSocket Reference"."OnStatusUpdated" format="%.0x"; "PLC boolean read Tags"."NVH Operator Sunshade Close Noise"."DataSocket Reference"."OnDataUpdated" format="%.0x"; "PLC boolean read Tags"."NVH Operator Sunshade Open Noise"."DataSocket Reference"."OnStatusUpdated" format="%.0x"; "PLC boolean read Tags"."NVH Operator Sunshade Open Noise"."DataSocket Reference"."OnDataUpdated" format="%.0x"; "PLC boolean read Tags"."NVH Operator Vent Close Noise"."DataSocket Reference"."OnStatusUpdated" format="%.0x"; "PLC boolean read Tags"."NVH Operator Vent Close Noise"."DataSocket Reference"."OnDataUpdated" format="%.0x"; "PLC boolean read Tags"."NVH Operator Vent Open Noise"."DataSocket Reference"."OnStatusUpdated" format="%.0x"; "PLC boolean read Tags"."NVH Operator Vent Open Noise"."DataSocket Reference"."OnDataUpdated" format="%.0x"; "PLC boolean read Tags"."NVH Operator Express Rollo Close02"."DataSocket Reference"."OnStatusUpdated" format="%.0x"; "PLC boolean read Tags"."NVH Operator Express Rollo Close02"."DataSocket Reference"."OnDataUpdated" format="%.0x"; "PLC boolean read Tags"."NVH Operator Express Rollo Open02"."DataSocket Reference"."OnStatusUpdated" format="%.0x"; "PLC boolean read Tags"."NVH Operator Express Rollo Open02"."DataSocket Reference"."OnDataUpdated" format="%.0x"; "PLC boolean read Tags"."NVH Operator Express Rollo Close01"."DataSocket Reference"."OnStatusUpdated" format="%.0x"; "PLC boolean read Tags"."NVH Operator Express Rollo Close01"."DataSocket Reference"."OnDataUpdated" format="%.0x"; "PLC boolean read Tags"."NVH Operator Express Rollo Open01"."DataSocket Reference"."OnStatusUpdated" format="%.0x"; "PLC boolean read Tags"."NVH Operator Express Rollo Open01"."DataSocket Reference"."OnDataUpdated" format="%.0x"; "PLC boolean read Tags"."NVH Operator Express Glass Close"."DataSocket Reference"."OnStatusUpdated" format="%.0x"; "PLC boolean read Tags"."NVH Operator Express Glass Close"."DataSocket Reference"."OnDataUpdated" format="%.0x"; "PLC boolean read Tags"."NVH Operator Express Glass Open"."DataSocket Reference"."OnStatusUpdated" format="%.0x"; "PLC boolean read Tags"."NVH Operator Express Glass Open"."DataSocket Reference"."OnDataUpdated" format="%.0x"; "PLC boolean read Tags"."NVH Operator Fail"."DataSocket Reference"."OnStatusUpdated" format="%.0x"; "PLC boolean read Tags"."NVH Operator Fail"."DataSocket Reference"."OnDataUpdated" format="%.0x"; "PLC boolean read Tags"."NVH Operator Pass"."DataSocket Reference"."OnStatusUpdated" format="%.0x"; "PLC boolean read Tags"."NVH Operator Pass"."DataSocket Reference"."OnDataUpdated" format="%.0x"; "PLC boolean read Tags"."Z LVDTs Extended"."DataSocket Reference"."OnStatusUpdated" format="%.0x"; "PLC boolean read Tags"."Z LVDTs Extended"."DataSocket Reference"."OnDataUpdated" format="%.0x"; "PLC boolean read Tags"."Check Frame Barcode"."DataSocket Reference"."OnStatusUpdated" format="%.0x"; "PLC boolean read Tags"."Check Frame Barcode"."DataSocket Reference"."OnDataUpdated" format="%.0x"; "PLC boolean read Tags"."SS Barcode Scanner Bypassed"."DataSocket Reference"."OnStatusUpdated" format="%.0x"; "PLC boolean read Tags"."SS Barcode Scanner Bypassed"."DataSocket Reference"."OnDataUpdated" format="%.0x"; "PLC boolean read Tags"."AT VentPMACisExtend"."DataSocket Reference"."OnStatusUpdated" format="%.0x"; "PLC boolean read Tags"."AT VentPMACisExtend"."DataSocket Reference"."OnDataUpdated" format="%.0x"; "PLC boolean read Tags"."AT VentPMACatHome"."DataSocket Reference"."OnStatusUpdated" format="%.0x"; "PLC boolean read Tags"."AT VentPMACatHome"."DataSocket Reference"."OnDataUpdated" format="%.0x"; "PLC boolean read Tags"."wind deflector low speed pos"."DataSocket Reference"."OnStatusUpdated" format="%.0x"; "PLC boolean read Tags"."wind deflector low speed pos"."DataSocket Reference"."OnDataUpdated" format="%.0x"; "PLC boolean read Tags"."wind deflector high speed pos"."DataSocket Reference"."OnStatusUpdated" format="%.0x"; "PLC boolean read Tags"."wind deflector high speed pos"."DataSocket Reference"."OnDataUpdated" format="%.0x"; "PLC boolean read Tags"."control slide right over stroke"."DataSocket Reference"."OnStatusUpdated" format="%.0x"; "PLC boolean read Tags"."control slide right over stroke"."DataSocket Reference"."OnDataUpdated" format="%.0x"; "PLC boolean read Tags"."control slide right good"."DataSocket Reference"."OnStatusUpdated" format="%.0x"; "PLC boolean read Tags"."control slide right good"."DataSocket Reference"."OnDataUpdated" format="%.0x"; "PLC boolean read Tags"."control slide left over stroke"."DataSocket Reference"."OnStatusUpdated" format="%.0x"; "PLC boolean read Tags"."control slide left over stroke"."DataSocket Reference"."OnDataUpdated" format="%.0x"; "PLC boolean read Tags"."control slide left good"."DataSocket Reference"."OnStatusUpdated" format="%.0x"; "PLC boolean read Tags"."control slide left good"."DataSocket Reference"."OnDataUpdated" format="%.0x"; "PLC boolean read Tags"."control slide at home"."DataSocket Reference"."OnStatusUpdated" format="%.0x"; "PLC boolean read Tags"."control slide at home"."DataSocket Reference"."OnDataUpdated" format="%.0x"; "PLC boolean read Tags"."ss servo closing"."DataSocket Reference"."OnStatusUpdated" format="%.0x"; "PLC boolean read Tags"."ss servo closing"."DataSocket Reference"."OnDataUpdated" format="%.0x"; "PLC boolean read Tags"."ss servo opening"."DataSocket Reference"."OnStatusUpdated" format="%.0x"; "PLC boolean read Tags"."ss servo opening"."DataSocket Reference"."OnDataUpdated" format="%.0x"; "PLC boolean read Tags"."ss servo at close"."DataSocket Reference"."OnStatusUpdated" format="%.0x"; "PLC boolean read Tags"."ss servo at close"."DataSocket Reference"."OnDataUpdated" format="%.0x"; "PLC boolean read Tags"."ss servo at open"."DataSocket Reference"."OnStatusUpdated" format="%.0x"; "PLC boolean read Tags"."ss servo at open"."DataSocket Reference"."OnDataUpdated" format="%.0x"; "PLC boolean read Tags"."manual barcode print"."DataSocket Reference"."OnStatusUpdated" format="%.0x"; "PLC boolean read Tags"."manual barcode print"."DataSocket Reference"."OnDataUpdated" format="%.0x"; "PLC boolean read Tags"."LVDT's Retracted"."DataSocket Reference"."OnStatusUpdated" format="%.0x"; "PLC boolean read Tags"."LVDT's Retracted"."DataSocket Reference"."OnDataUpdated" format="%.0x"; "PLC boolean read Tags"."abort"."DataSocket Reference"."OnStatusUpdated" format="%.0x"; "PLC boolean read Tags"."abort"."DataSocket Reference"."OnDataUpdated" format="%.0x"; "PLC boolean read Tags"."start"."DataSocket Reference"."OnStatusUpdated" format="%.0x"; "PLC boolean read Tags"."start"."DataSocket Reference"."OnDataUpdated" format="%.0x"; "PLC boolean read Tags"."bolt check 8"."DataSocket Reference"."OnStatusUpdated" format="%.0x"; "PLC boolean read Tags"."bolt check 8"."DataSocket Reference"."OnDataUpdated" format="%.0x"; "PLC boolean read Tags"."bolt check 7"."DataSocket Reference"."OnStatusUpdated" format="%.0x"; "PLC boolean read Tags"."bolt check 7"."DataSocket Reference"."OnDataUpdated" format="%.0x"; "PLC boolean read Tags"."bolt check 6"."DataSocket Reference"."OnStatusUpdated" format="%.0x"; "PLC boolean read Tags"."bolt check 6"."DataSocket Reference"."OnDataUpdated" format="%.0x"; "PLC boolean read Tags"."bolt check 5"."DataSocket Reference"."OnStatusUpdated" format="%.0x"; "PLC boolean read Tags"."bolt check 5"."DataSocket Reference"."OnDataUpdated" format="%.0x"; "PLC boolean read Tags"."bolt check 4"."DataSocket Reference"."OnStatusUpdated" format="%.0x"; "PLC boolean read Tags"."bolt check 4"."DataSocket Reference"."OnDataUpdated" format="%.0x"; "PLC boolean read Tags"."bolt check 3"."DataSocket Reference"."OnStatusUpdated" format="%.0x"; "PLC boolean read Tags"."bolt check 3"."DataSocket Reference"."OnDataUpdated" format="%.0x"; "PLC boolean read Tags"."bolt check 2"."DataSocket Reference"."OnStatusUpdated" format="%.0x"; "PLC boolean read Tags"."bolt check 2"."DataSocket Reference"."OnDataUpdated" format="%.0x"; "PLC boolean read Tags"."bolt check 1"."DataSocket Reference"."OnStatusUpdated" format="%.0x"; "PLC boolean read Tags"."bolt check 1"."DataSocket Reference"."OnDataUpdated" format="%.0x"; "PLC boolean read Tags"."LVDT's Extended"."DataSocket Reference"."OnStatusUpdated" format="%.0x"; "PLC boolean read Tags"."LVDT's Extended"."DataSocket Reference"."OnDataUpdated" format="%.0x"; "PLC boolean read Tags"."AT in wand home pos"."DataSocket Reference"."OnStatusUpdated" format="%.0x"; "PLC boolean read Tags"."AT in wand home pos"."DataSocket Reference"."OnDataUpdated" format="%.0x"; "PLC boolean read Tags"."AT in sunshad wand lower pos"."DataSocket Reference"."OnStatusUpdated" format="%.0x"; "PLC boolean read Tags"."AT in sunshad wand lower pos"."DataSocket Reference"."OnDataUpdated" format="%.0x"; "PLC boolean read Tags"."AT in glass wand lower pos"."DataSocket Reference"."OnStatusUpdated" format="%.0x"; "PLC boolean read Tags"."AT in glass wand lower pos"."DataSocket Reference"."OnDataUpdated" format="%.0x"; "PLC boolean read Tags"."AT shade position"."DataSocket Reference"."OnStatusUpdated" format="%.0x"; "PLC boolean read Tags"."AT shade position"."DataSocket Reference"."OnDataUpdated" format="%.0x"; "PLC boolean read Tags"."AT glass position"."DataSocket Reference"."OnStatusUpdated" format="%.0x"; "PLC boolean read Tags"."AT glass position"."DataSocket Reference"."OnDataUpdated" format="%.0x"}, 2 "ok?":bool, 3 "Config Info out":variant)   [LabVIEW 2018]
uses:
  Type Def's/Config Info.ctl
  02.Type Def's/plc comms params.ctl
  02.Type Def's/station plc read boolean tags.ctl
  05.UserVI's/type defs/plc path and tag.ctl
  <vilib>/Platform/dataskt.llb/DataSocket Reference Type.ctl
  02.Type Def's/station plc write boolean tags.ctl
  02.Type Def's/station plc read string tags.ctl
  02.Type Def's/station plc write string tags.ctl
panel:
  # "start/abort only used by barcode instance, since there are discrete signals for this in the other stations."
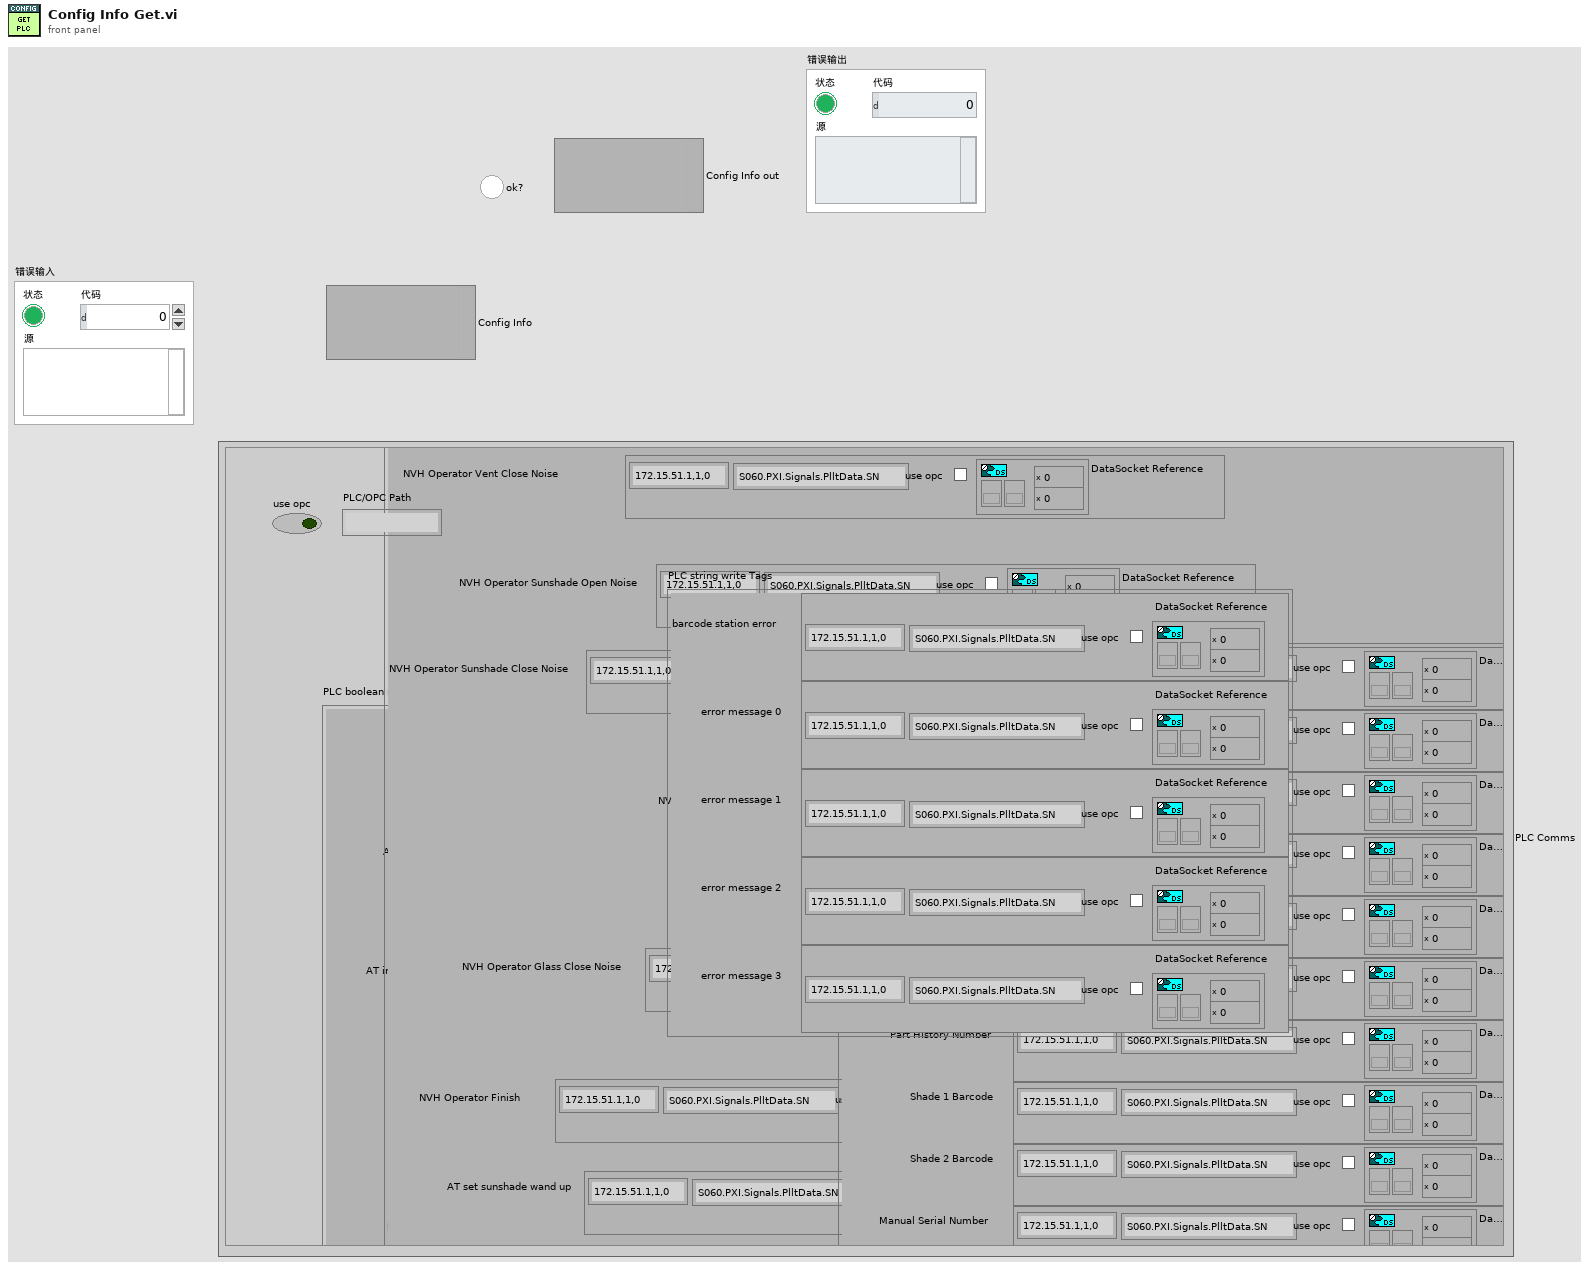
[diagram p1: front panel]
types:
  T1 = typedef "plc comms params.ctl" = cluster{"PLC boolean read Tags":T2, "PLC bool write Tags":T5, "PLC string read Tags":T6, "PLC string write Tags":T7, "use opc":bool, "PLC/OPC Path":string}
  T2 = typedef "station plc read boolean tags.ctl" = cluster{"AT glass position":T3, "AT shade position":T3, "AT in glass wand lower pos":T3, "AT in glass wand up pos":T3, "AT in sunshad wand lower pos":T3, "AT in sunshad wand up pos":T3, "AT in wand home pos":T3, "LVDT's Extended":T3, "bolt check 1":T3, "bolt check 2":T3, "bolt check 3":T3, "bolt check 4":T3, "bolt check 5":T3, "bolt check 6":T3, "bolt check 7":T3, "bolt check 8":T3, "start":T3, "abort":T3, "LVDT's Retracted":T3, "manual barcode print":T3, "ss servo at open":T3, "ss servo at close":T3, "ss servo opening":T3, "ss servo closing":T3, "control slide at home":T3, "control slide left good":T3, "control slide left over stroke":T3, "control slide right good":T3, "control slide right over stroke":T3, "wind deflector high speed pos":T3, "wind deflector low speed pos":T3, "AT VentPMACatHome":T3, "AT VentPMACisExtend":T3, "SS Barcode Scanner Bypassed":T3, "Check Frame Barcode":T3, "Z LVDTs Extended":T3, "NVH Operator Pass":T3, "NVH Operator Fail":T3, "NVH Operator Express Glass Open":T3, "NVH Operator Express Glass Close":T3, "NVH Operator Express Rollo Open01":T3, "NVH Operator Express Rollo Close01":T3, "NVH Operator Express Rollo Open02":T3, "NVH Operator Express Rollo Close02":T3, "NVH Operator Vent Open Noise":T3, "NVH Operator Vent Close Noise":T3, "NVH Operator Sunshade Open Noise":T3, "NVH Operator Sunshade Close Noise":T3, "NVH Operator Glass Open Noise":T3, "NVH Operator Glass Close Noise":T3, "NVH Operator Finish":T3, "NVH Operator Check":T3, "windproof position":T3, "NVH Operator Express Glass vent Open":T3, "NVH Operator Express Glass Vent Close":T3, "NVH Operator Re-do":T3, "AT at vent ATS test pos":T3, "AT at vent ATS Home pos":T3, "Start Adjust LVDT":T3, "Finish Adjust LVDT":T3}
  T3 = typedef "plc path and tag.ctl" = cluster{"Tag Name":string, "Network Path":string, "use opc":bool, "DataSocket Reference":T4}
  T4 = typedef "DataSocket Reference Type.ctl" = cluster{"CWDSLib._DCWDataSocket":refnum<k7>, "CWDSLib._DCWData":refnum<k7>, "OnDataUpdated":u32, "OnStatusUpdated":u32}
  T5 = typedef "station plc write boolean tags.ctl" = cluster{"AT set glass wand lower":T3, "AT set sunshade wand lower":T3, "AT set sunshade wand up":T3, "AT set glass wand up":T3, "AT set wand home pos":T3, "Test Complete Pass":T3, "Test Complete Fail":T3, "Test Started":T3, "Retract LVDT's":T3, "Extend LVDT's":T3, "ss servo open":T3, "ss servo close":T3, "control slide start":T3, "control slide stop":T3, "AT VentPMACHome":T3, "AT VentPMACExtended":T3, "Good Frame Barcode":T3, "Bad Frame Barcode":T3, "Extend Z LVDTS":T3, "NVH SunRoof Moving":T3, "NVH SunRoof Stop":T3, "NVH Pass":T3, "NVH Fail":T3, "NVH Operator Express Glass Opened":T3, "NVH Operator Express Glass Closed":T3, "NVH Operator Express Rollo Opened01":T3, "NVH Operator Express Rollo Closed01":T3, "NVH Operator Express Rollo Opened02":T3, "NVH Operator Pass":T3, "NVH Operator Fail":T3, "NVH Operator Check":T3, "NVH Operator Vent Open Noise":T3, "NVH Operator Vent Close Noise":T3, "NVH Operator Sunshade Open Noise":T3, "NVH Operator Sunshade Close Noise":T3, "NVH Operator Glass Open Noise":T3, "NVH Operator Glass Close Noise":T3, "NVH Operator Finish":T3, "Barcode01 OK":T3, "Barcode02 OK":T3, "AT set to Vent ATS Test Pos":T3, "AT set to Vent ATS Home Pos":T3, "Move LVDT Adjust Station":T3}
  T6 = typedef "station plc read string tags.ctl" = cluster{"Serial Number":T3, "Pallet Number":T3, "Inalfa Part Number":T3, "Shade Color":T3, "Model Type":T3, "Customer Number":T3, "Part History Number":T3, "Shade 1 Barcode":T3, "Shade 2 Barcode":T3, "Manual Serial Number":T3, "Manual Inalfa Part Number":T3, "Manual Shade Color":T3, "Manual Model Type":T3, "Manual Customer Number":T3, "Manual Part History Number":T3}
  T7 = typedef "station plc write string tags.ctl" = cluster{"barcode station error":T3, "error message 0":T3, "error message 1":T3, "error message 2":T3, "error message 3":T3}
  T8 = typedef "Config Info.ctl" = variant
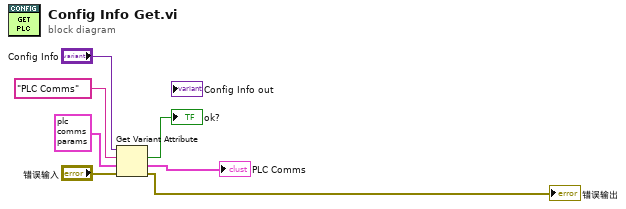
[diagram p0: block diagram]
diagram:
  n1 = Get Variant Attribute(Variant="Config Info", name="PLC Comms" ("名称"), default value (empty Variant)=T1 {"PLC boolean read Tags"={"AT glass position"={"Tag Name"="S060.PXI.Signals.PlltData.SN", "Network Path"="172.15.51.1,1,0", "use opc"=FALSE, "DataSocket Reference"={"CWDSLib._DCWDataSocket"=refnum, "CWDSLib._DCWData"=refnum, "OnDataUpdated"=0, "OnStatusUpdated"=0}}, "AT shade position"={"Tag Name"="S060.PXI.Signals.PlltData.SN", "Network Path"="172.15.51.1,1,0", "use opc"=FALSE, "DataSocket Reference"={"CWDSLib._DCWDataSocket"=refnum, "CWDSLib._DCWData"=refnum, "OnDataUpdated"=0, "OnStatusUpdated"=0}}, "AT in glass wand lower pos"={"Tag Name"="S060.PXI.Signals.PlltData.SN", "Network Path"="172.15.51.1,1,0", "use opc"=FALSE, "DataSocket Reference"={"CWDSLib._DCWDataSocket"=refnum, "CWDSLib._DCWData"=refnum, "OnDataUpdated"=0, "OnStatusUpdated"=0}}, "AT in glass wand up pos"={"Tag Name"="S060.PXI.Signals.PlltData.SN", "Network Path"="172.15.51.1,1,0", "use opc"=FALSE, "DataSocket Reference"={"CWDSLib._DCWDataSocket"=refnum, "CWDSLib._DCWData"=refnum, "OnDataUpdated"=0, "OnStatusUpdated"=0}}, "AT in sunshad wand lower pos"={"Tag Name"="S060.PXI.Signals.PlltData.SN", "Network Path"="172.15.51.1,1,0", "use opc"=FALSE, "DataSocket Reference"={"CWDSLib._DCWDataSocket"=refnum, "CWDSLib._DCWData"=refnum, "OnDataUpdated"=0, "OnStatusUpdated"=0}}, "AT in sunshad wand up pos"={"Tag Name"="S060.PXI.Signals.PlltData.SN", "Network Path"="172.15.51.1,1,0", "use opc"=FALSE, "DataSocket Reference"={"CWDSLib._DCWDataSocket"=refnum, "CWDSLib._DCWData"=refnum, "OnDataUpdated"=0, "OnStatusUpdated"=0}}, "AT in wand home pos"={"Tag Name"="S060.PXI.Signals.PlltData.SN", "Network Path"="172.15.51.1,1,0", "use opc"=FALSE, "DataSocket Reference"={"CWDSLib._DCWDataSocket"=refnum, "CWDSLib._DCWData"=refnum, "OnDataUpdated"=0, "OnStatusUpdated"=0}}, "LVDT's Extended"={"Tag Name"="S060.PXI.Signals.PlltData.SN", "Network Path"="172.15.51.1,1,0", "use opc"=FALSE, "DataSocket Reference"={"CWDSLib._DCWDataSocket"=refnum, "CWDSLib._DCWData"=refnum, "OnDataUpdated"=0, "OnStatusUpdated"=0}}, "bolt check 1"={"Tag Name"="S060.PXI.Signals.PlltData.SN", "Network Path"="172.15.51.1,1,0", "use opc"=FALSE, "DataSocket Reference"={"CWDSLib._DCWDataSocket"=refnum, "CWDSLib._DCWData"=refnum, "OnDataUpdated"=0, "OnStatusUpdated"=0}}, "bolt check 2"={"Tag Name"="S060.PXI.Signals.PlltData.SN", "Network Path"="172.15.51.1,1,0", "use opc"=FALSE, "DataSocket Reference"={"CWDSLib._DCWDataSocket"=refnum, "CWDSLib._DCWData"=refnum, "OnDataUpdated"=0, "OnStatusUpdated"=0}}, "bolt check 3"={"Tag Name"="S060.PXI.Signals.PlltData.SN", "Network Path"="172.15.51.1,1,0", "use opc"=FALSE, "DataSocket Reference"={"CWDSLib._DCWDataSocket"=refnum, "CWDSLib._DCWData"=refnum, "OnDataUpdated"=0, "OnStatusUpdated"=0}}, "bolt check 4"={"Tag Name"="S060.PXI.Signals.PlltData.SN", "Network Path"="172.15.51.1,1,0", "use opc"=FALSE, "DataSocket Reference"={"CWDSLib._DCWDataSocket"=refnum, "CWDSLib._DCWData"=refnum, "OnDataUpdated"=0, "OnStatusUpdated"=0}}, "bolt check 5"={"Tag Name"="S060.PXI.Signals.PlltData.SN", "Network Path"="172.15.51.1,1,0", "use opc"=FALSE, "DataSocket Reference"={"CWDSLib._DCWDataSocket"=refnum, "CWDSLib._DCWData"=refnum, "OnDataUpdated"=0, "OnStatusUpdated"=0}}, "bolt check 6"={"Tag Name"="S060.PXI.Signals.PlltData.SN", "Network Path"="172.15.51.1,1,0", "use opc"=FALSE, "DataSocket Reference"={"CWDSLib._DCWDataSocket"=refnum, "CWDSLib._DCWData"=refnum, "OnDataUpdated"=0, "OnStatusUpdated"=0}}, "bolt check 7"={"Tag Name"="S060.PXI.Signals.PlltData.SN", "Network Path"="172.15.51.1,1,0", "use opc"=FALSE, "DataSocket Reference"={"CWDSLib._DCWDataSocket"=refnum, "CWDSLib._DCWData"=refnum, "OnDataUpdated"=0, "OnStatusUpdated"=0}}, "bolt check 8"={"Tag Name"="S060.PXI.Signals.PlltData.SN", "Network Path"="172.15.51.1,1,0", "use opc"=FALSE, "DataSocket Reference"={"CWDSLib._DCWDataSocket"=refnum, "CWDSLib._DCWData"=refnum, "OnDataUpdated"=0, "OnStatusUpdated"=0}}, "start"={"Tag Name"="S060.PXI.Signals.PlltData.SN", "Network Path"="172.15.51.1,1,0", "use opc"=FALSE, "DataSocket Reference"={"CWDSLib._DCWDataSocket"=refnum, "CWDSLib._DCWData"=refnum, "OnDataUpdated"=0, "OnStatusUpdated"=0}}, "abort"={"Tag Name"="S060.PXI.Signals.PlltData.SN", "Network Path"="172.15.51.1,1,0", "use opc"=FALSE, "DataSocket Reference"={"CWDSLib._DCWDataSocket"=refnum, "CWDSLib._DCWData"=refnum, "OnDataUpdated"=0, "OnStatusUpdated"=0}}, "LVDT's Retracted"={"Tag Name"="S060.PXI.Signals.PlltData.SN", "Network Path"="172.15.51.1,1,0", "use opc"=FALSE, "DataSocket Reference"={"CWDSLib._DCWDataSocket"=refnum, "CWDSLib._DCWData"=refnum, "OnDataUpdated"=0, "OnStatusUpdated"=0}}, "manual barcode print"={"Tag Name"="S060.PXI.Signals.PlltData.SN", "Network Path"="172.15.51.1,1,0", "use opc"=FALSE, "DataSocket Reference"={"CWDSLib._DCWDataSocket"=refnum, "CWDSLib._DCWData"=refnum, "OnDataUpdated"=0, "OnStatusUpdated"=0}}, "ss servo at open"={"Tag Name"="S060.PXI.Signals.PlltData.SN", "Network Path"="172.15.51.1,1,0", "use opc"=FALSE, "DataSocket Reference"={"CWDSLib._DCWDataSocket"=refnum, "CWDSLib._DCWData"=refnum, "OnDataUpdated"=0, "OnStatusUpdated"=0}}, "ss servo at close"={"Tag Name"="S060.PXI.Signals.PlltData.SN", "Network Path"="172.15.51.1,1,0", "use opc"=FALSE, "DataSocket Reference"={"CWDSLib._DCWDataSocket"=refnum, "CWDSLib._DCWData"=refnum, "OnDataUpdated"=0, "OnStatusUpdated"=0}}, "ss servo opening"={"Tag Name"="S060.PXI.Signals.PlltData.SN", "Network Path"="172.15.51.1,1,0", "use opc"=FALSE, "DataSocket Reference"={"CWDSLib._DCWDataSocket"=refnum, "CWDSLib._DCWData"=refnum, "OnDataUpdated"=0, "OnStatusUpdated"=0}}, "ss servo closing"={"Tag Name"="S060.PXI.Signals.PlltData.SN", "Network Path"="172.15.51.1,1,0", "use opc"=FALSE, "DataSocket Reference"={"CWDSLib._DCWDataSocket"=refnum, "CWDSLib._DCWData"=refnum, "OnDataUpdated"=0, "OnStatusUpdated"=0}}, "control slide at home"={"Tag Name"="S060.PXI.Signals.PlltData.SN", "Network Path"="172.15.51.1,1,0", "use opc"=FALSE, "DataSocket Reference"={"CWDSLib._DCWDataSocket"=refnum, "CWDSLib._DCWData"=refnum, "OnDataUpdated"=0, "OnStatusUpdated"=0}}, "control slide left good"={"Tag Name"="S060.PXI.Signals.PlltData.SN", "Network Path"="172.15.51.1,1,0", "use opc"=FALSE, "DataSocket Reference"={"CWDSLib._DCWDataSocket"=refnum, "CWDSLib._DCWData"=refnum, "OnDataUpdated"=0, "OnStatusUpdated"=0}}, "control slide left over stroke"={"Tag Name"="S060.PXI.Signals.PlltData.SN", "Network Path"="172.15.51.1,1,0", "use opc"=FALSE, "DataSocket Reference"={"CWDSLib._DCWDataSocket"=refnum, "CWDSLib._DCWData"=refnum, "OnDataUpdated"=0, "OnStatusUpdated"=0}}, "control slide right good"={"Tag Name"="S060.PXI.Signals.PlltData.SN", "Network Path"="172.15.51.1,1,0", "use opc"=FALSE, "DataSocket Reference"={"CWDSLib._DCWDataSocket"=refnum, "CWDSLib._DCWData"=refnum, "OnDataUpdated"=0, "OnStatusUpdated"=0}}, "control slide right over stroke"={"Tag Name"="S060.PXI.Signals.PlltData.SN", "Network Path"="172.15.51.1,1,0", "use opc"=FALSE, "DataSocket Reference"={"CWDSLib._DCWDataSocket"=refnum, "CWDSLib._DCWData"=refnum, "OnDataUpdated"=0, "OnStatusUpdated"=0}}, "wind deflector high speed pos"={"Tag Name"="S060.PXI.Signals.PlltData.SN", "Network Path"="172.15.51.1,1,0", "use opc"=FALSE, "DataSocket Reference"={"CWDSLib._DCWDataSocket"=refnum, "CWDSLib._DCWData"=refnum, "OnDataUpdated"=0, "OnStatusUpdated"=0}}, "wind deflector low speed pos"={"Tag Name"="S060.PXI.Signals.PlltData.SN", "Network Path"="172.15.51.1,1,0", "use opc"=FALSE, "DataSocket Reference"={"CWDSLib._DCWDataSocket"=refnum, "CWDSLib._DCWData"=refnum, "OnDataUpdated"=0, "OnStatusUpdated"=0}}, "AT VentPMACatHome"={"Tag Name"="S060.PXI.Signals.PlltData.SN", "Network Path"="172.15.51.1,1,0", "use opc"=FALSE, "DataSocket Reference"={"CWDSLib._DCWDataSocket"=refnum, "CWDSLib._DCWData"=refnum, "OnDataUpdated"=0, "OnStatusUpdated"=0}}, "AT VentPMACisExtend"={"Tag Name"="S060.PXI.Signals.PlltData.SN", "Network Path"="172.15.51.1,1,0", "use opc"=FALSE, "DataSocket Reference"={"CWDSLib._DCWDataSocket"=refnum, "CWDSLib._DCWData"=refnum, "OnDataUpdated"=0, "OnStatusUpdated"=0}}, "SS Barcode Scanner Bypassed"={"Tag Name"="S060.PXI.Signals.PlltData.SN", "Network Path"="172.15.51.1,1,0", "use opc"=FALSE, "DataSocket Reference"={"CWDSLib._DCWDataSocket"=refnum, "CWDSLib._DCWData"=refnum, "OnDataUpdated"=0, "OnStatusUpdated"=0}}, "Check Frame Barcode"={"Tag Name"="S060.PXI.Signals.PlltData.SN", "Network Path"="172.15.51.1,1,0", "use opc"=FALSE, "DataSocket Reference"={"CWDSLib._DCWDataSocket"=refnum, "CWDSLib._DCWData"=refnum, "OnDataUpdated"=0, "OnStatusUpdated"=0}}, "Z LVDTs Extended"={"Tag Name"="S060.PXI.Signals.PlltData.SN", "Network Path"="172.15.51.1,1,0", "use opc"=FALSE, "DataSocket Reference"={"CWDSLib._DCWDataSocket"=refnum, "CWDSLib._DCWData"=refnum, "OnDataUpdated"=0, "OnStatusUpdated"=0}}, "NVH Operator Pass"={"Tag Name"="S060.PXI.Signals.PlltData.SN", "Network Path"="172.15.51.1,1,0", "use opc"=FALSE, "DataSocket Reference"={"CWDSLib._DCWDataSocket"=refnum, "CWDSLib._DCWData"=refnum, "OnDataUpdated"=0, "OnStatusUpdated"=0}}, "NVH Operator Fail"={"Tag Name"="S060.PXI.Signals.PlltData.SN", "Network Path"="172.15.51.1,1,0", "use opc"=FALSE, "DataSocket Reference"={"CWDSLib._DCWDataSocket"=refnum, "CWDSLib._DCWData"=refnum, "OnDataUpdated"=0, "OnStatusUpdated"=0}}, "NVH Operator Express Glass Open"={"Tag Name"="S060.PXI.Signals.PlltData.SN", "Network Path"="172.15.51.1,1,0", "use opc"=FALSE, "DataSocket Reference"={"CWDSLib._DCWDataSocket"=refnum, "CWDSLib._DCWData"=refnum, "OnDataUpdated"=0, "OnStatusUpdated"=0}}, "NVH Operator Express Glass Close"={"Tag Name"="S060.PXI.Signals.PlltData.SN", "Network Path"="172.15.51.1,1,0", "use opc"=FALSE, "DataSocket Reference"={"CWDSLib._DCWDataSocket"=refnum, "CWDSLib._DCWData"=refnum, "OnDataUpdated"=0, "OnStatusUpdated"=0}}, "NVH Operator Express Rollo Open01"={"Tag Name"="S060.PXI.Signals.PlltData.SN", "Network Path"="172.15.51.1,1,0", "use opc"=FALSE, "DataSocket Reference"={"CWDSLib._DCWDataSocket"=refnum, "CWDSLib._DCWData"=refnum, "OnDataUpdated"=0, "OnStatusUpdated"=0}}, "NVH Operator Express Rollo Close01"={"Tag Name"="S060.PXI.Signals.PlltData.SN", "Network Path"="172.15.51.1,1,0", "use opc"=FALSE, "DataSocket Reference"={"CWDSLib._DCWDataSocket"=refnum, "CWDSLib._DCWData"=refnum, "OnDataUpdated"=0, "OnStatusUpdated"=0}}, "NVH Operator Express Rollo Open02"={"Tag Name"="S060.PXI.Signals.PlltData.SN", "Network Path"="172.15.51.1,1,0", "use opc"=FALSE, "DataSocket Reference"={"CWDSLib._DCWDataSocket"=refnum, "CWDSLib._DCWData"=refnum, "OnDataUpdated"=0, "OnStatusUpdated"=0}}, "NVH Operator Express Rollo Close02"={"Tag Name"="S060.PXI.Signals.PlltData.SN", "Network Path"="172.15.51.1,1,0", "use opc"=FALSE, "DataSocket Reference"={"CWDSLib._DCWDataSocket"=refnum, "CWDSLib._DCWData"=refnum, "OnDataUpdated"=0, "OnStatusUpdated"=0}}, "NVH Operator Vent Open Noise"={"Tag Name"="S060.PXI.Signals.PlltData.SN", "Network Path"="172.15.51.1,1,0", "use opc"=FALSE, "DataSocket Reference"={"CWDSLib._DCWDataSocket"=refnum, "CWDSLib._DCWData"=refnum, "OnDataUpdated"=0, "OnStatusUpdated"=0}}, "NVH Operator Vent Close Noise"={"Tag Name"="S060.PXI.Signals.PlltData.SN", "Network Path"="172.15.51.1,1,0", "use opc"=FALSE, "DataSocket Reference"={"CWDSLib._DCWDataSocket"=refnum, "CWDSLib._DCWData"=refnum, "OnDataUpdated"=0, "OnStatusUpdated"=0}}, "NVH Operator Sunshade Open Noise"={"Tag Name"="S060.PXI.Signals.PlltData.SN", "Network Path"="172.15.51.1,1,0", "use opc"=FALSE, "DataSocket Reference"={"CWDSLib._DCWDataSocket"=refnum, "CWDSLib._DCWData"=refnum, "OnDataUpdated"=0, "OnStatusUpdated"=0}}, "NVH Operator Sunshade Close Noise"={"Tag Name"="S060.PXI.Signals.PlltData.SN", "Network Path"="172.15.51.1,1,0", "use opc"=FALSE, "DataSocket Reference"={"CWDSLib._DCWDataSocket"=refnum, "CWDSLib._DCWData"=refnum, "OnDataUpdated"=0, "OnStatusUpdated"=0}}, "NVH Operator Glass Open Noise"={"Tag Name"="S060.PXI.Signals.PlltData.SN", "Network Path"="172.15.51.1,1,0", "use opc"=FALSE, "DataSocket Reference"={"CWDSLib._DCWDataSocket"=refnum, "CWDSLib._DCWData"=refnum, "OnDataUpdated"=0, "OnStatusUpdated"=0}}, "NVH Operator Glass Close Noise"={"Tag Name"="S060.PXI.Signals.PlltData.SN", "Network Path"="172.15.51.1,1,0", "use opc"=FALSE, "DataSocket Reference"={"CWDSLib._DCWDataSocket"=refnum, "CWDSLib._DCWData"=refnum, "OnDataUpdated"=0, "OnStatusUpdated"=0}}, "NVH Operator Finish"={"Tag Name"="S060.PXI.Signals.PlltData.SN", "Network Path"="172.15.51.1,1,0", "use opc"=FALSE, "DataSocket Reference"={"CWDSLib._DCWDataSocket"=refnum, "CWDSLib._DCWData"=refnum, "OnDataUpdated"=0, "OnStatusUpdated"=0}}, "NVH Operator Check"={"Tag Name"="S060.PXI.Signals.PlltData.SN", "Network Path"="172.15.51.1,1,0", "use opc"=FALSE, "DataSocket Reference"={"CWDSLib._DCWDataSocket"=refnum, "CWDSLib._DCWData"=refnum, "OnDataUpdated"=0, "OnStatusUpdated"=0}}, "windproof position"={"Tag Name"="S060.PXI.Signals.PlltData.SN", "Network Path"="172.15.51.1,1,0", "use opc"=FALSE, "DataSocket Reference"={"CWDSLib._DCWDataSocket"=refnum, "CWDSLib._DCWData"=refnum, "OnDataUpdated"=0, "OnStatusUpdated"=0}}, "NVH Operator Express Glass vent Open"={"Tag Name"="S060.PXI.Signals.PlltData.SN", "Network Path"="172.15.51.1,1,0", "use opc"=FALSE, "DataSocket Reference"={"CWDSLib._DCWDataSocket"=refnum, "CWDSLib._DCWData"=refnum, "OnDataUpdated"=0, "OnStatusUpdated"=0}}, "NVH Operator Express Glass Vent Close"={"Tag Name"="S060.PXI.Signals.PlltData.SN", "Network Path"="172.15.51.1,1,0", "use opc"=FALSE, "DataSocket Reference"={"CWDSLib._DCWDataSocket"=refnum, "CWDSLib._DCWData"=refnum, "OnDataUpdated"=0, "OnStatusUpdated"=0}}, "NVH Operator Re-do"={"Tag Name"="S060.PXI.Signals.PlltData.SN", "Network Path"="172.15.51.1,1,0", "use opc"=FALSE, "DataSocket Reference"={"CWDSLib._DCWDataSocket"=refnum, "CWDSLib._DCWData"=refnum, "OnDataUpdated"=0, "OnStatusUpdated"=0}}, "AT at vent ATS test pos"={"Tag Name"="S060.PXI.Signals.PlltData.SN", "Network Path"="172.15.51.1,1,0", "use opc"=FALSE, "DataSocket Reference"={"CWDSLib._DCWDataSocket"=refnum, "CWDSLib._DCWData"=refnum, "OnDataUpdated"=0, "OnStatusUpdated"=0}}, "AT at vent ATS Home pos"={"Tag Name"="S060.PXI.Signals.PlltData.SN", "Network Path"="172.15.51.1,1,0", "use opc"=FALSE, "DataSocket Reference"={"CWDSLib._DCWDataSocket"=refnum, "CWDSLib._DCWData"=refnum, "OnDataUpdated"=0, "OnStatusUpdated"=0}}, "Start Adjust LVDT"={"Tag Name"="S060.PXI.Signals.PlltData.SN", "Network Path"="172.15.51.1,1,0", "use opc"=FALSE, "DataSocket Reference"={"CWDSLib._DCWDataSocket"=refnum, "CWDSLib._DCWData"=refnum, "OnDataUpdated"=0, "OnStatusUpdated"=0}}, "Finish Adjust LVDT"={"Tag Name"="S060.PXI.Signals.PlltData.SN", "Network Path"="172.15.51.1,1,0", "use opc"=FALSE, "DataSocket Reference"={"CWDSLib._DCWDataSocket"=refnum, "CWDSLib._DCWData"=refnum, "OnDataUpdated"=0, "OnStatusUpdated"=0}}}, "PLC bool write Tags"={"AT set glass wand lower"={"Tag Name"="S060.PXI.Signals.PlltData.SN", "Network Path"="172.15.51.1,1,0", "use opc"=FALSE, "DataSocket Reference"={"CWDSLib._DCWDataSocket"=refnum, "CWDSLib._DCWData"=refnum, "OnDataUpdated"=0, "OnStatusUpdated"=0}}, "AT set sunshade wand lower"={"Tag Name"="S060.PXI.Signals.PlltData.SN", "Network Path"="172.15.51.1,1,0", "use opc"=FALSE, "DataSocket Reference"={"CWDSLib._DCWDataSocket"=refnum, "CWDSLib._DCWData"=refnum, "OnDataUpdated"=0, "OnStatusUpdated"=0}}, "AT set sunshade wand up"={"Tag Name"="S060.PXI.Signals.PlltData.SN", "Network Path"="172.15.51.1,1,0", "use opc"=FALSE, "DataSocket Reference"={"CWDSLib._DCWDataSocket"=refnum, "CWDSLib._DCWData"=refnum, "OnDataUpdated"=0, "OnStatusUpdated"=0}}, "AT set glass wand up"={"Tag Name"="S060.PXI.Signals.PlltData.SN", "Network Path"="172.15.51.1,1,0", "use opc"=FALSE, "DataSocket Reference"={"CWDSLib._DCWDataSocket"=refnum, "CWDSLib._DCWData"=refnum, "OnDataUpdated"=0, "OnStatusUpdated"=0}}, "AT set wand home pos"={"Tag Name"="S060.PXI.Signals.PlltData.SN", "Network Path"="172.15.51.1,1,0", "use opc"=FALSE, "DataSocket Reference"={"CWDSLib._DCWDataSocket"=refnum, "CWDSLib._DCWData"=refnum, "OnDataUpdated"=0, "OnStatusUpdated"=0}}, "Test Complete Pass"={"Tag Name"="S060.PXI.Signals.PlltData.SN", "Network Path"="172.15.51.1,1,0", "use opc"=FALSE, "DataSocket Reference"={"CWDSLib._DCWDataSocket"=refnum, "CWDSLib._DCWData"=refnum, "OnDataUpdated"=0, "OnStatusUpdated"=0}}, "Test Complete Fail"={"Tag Name"="S060.PXI.Signals.PlltData.SN", "Network Path"="172.15.51.1,1,0", "use opc"=FALSE, "DataSocket Reference"={"CWDSLib._DCWDataSocket"=refnum, "CWDSLib._DCWData"=refnum, "OnDataUpdated"=0, "OnStatusUpdated"=0}}, "Test Started"={"Tag Name"="S060.PXI.Signals.PlltData.SN", "Network Path"="172.15.51.1,1,0", "use opc"=FALSE, "DataSocket Reference"={"CWDSLib._DCWDataSocket"=refnum, "CWDSLib._DCWData"=refnum, "OnDataUpdated"=0, "OnStatusUpdated"=0}}, "Retract LVDT's"={"Tag Name"="S060.PXI.Signals.PlltData.SN", "Network Path"="172.15.51.1,1,0", "use opc"=FALSE, "DataSocket Reference"={"CWDSLib._DCWDataSocket"=refnum, "CWDSLib._DCWData"=refnum, "OnDataUpdated"=0, "OnStatusUpdated"=0}}, "Extend LVDT's"={"Tag Name"="S060.PXI.Signals.PlltData.SN", "Network Path"="172.15.51.1,1,0", "use opc"=FALSE, "DataSocket Reference"={"CWDSLib._DCWDataSocket"=refnum, "CWDSLib._DCWData"=refnum, "OnDataUpdated"=0, "OnStatusUpdated"=0}}, "ss servo open"={"Tag Name"="S060.PXI.Signals.PlltData.SN", "Network Path"="172.15.51.1,1,0", "use opc"=FALSE, "DataSocket Reference"={"CWDSLib._DCWDataSocket"=refnum, "CWDSLib._DCWData"=refnum, "OnDataUpdated"=0, "OnStatusUpdated"=0}}, "ss servo close"={"Tag Name"="S060.PXI.Signals.PlltData.SN", "Network Path"="172.15.51.1,1,0", "use opc"=FALSE, "DataSocket Reference"={"CWDSLib._DCWDataSocket"=refnum, "CWDSLib._DCWData"=refnum, "OnDataUpdated"=0, "OnStatusUpdated"=0}}, "control slide start"={"Tag Name"="S060.PXI.Signals.PlltData.SN", "Network Path"="172.15.51.1,1,0", "use opc"=FALSE, "DataSocket Reference"={"CWDSLib._DCWDataSocket"=refnum, "CWDSLib._DCWData"=refnum, "OnDataUpdated"=0, "OnStatusUpdated"=0}}, "control slide stop"={"Tag Name"="S060.PXI.Signals.PlltData.SN", "Network Path"="172.15.51.1,1,0", "use opc"=FALSE, "DataSocket Reference"={"CWDSLib._DCWDataSocket"=refnum, "CWDSLib._DCWData"=refnum, "OnDataUpdated"=0, "OnStatusUpdated"=0}}, "AT VentPMACHome"={"Tag Name"="S060.PXI.Signals.PlltData.SN", "Network Path"="172.15.51.1,1,0", "use opc"=FALSE, "DataSocket Reference"={"CWDSLib._DCWDataSocket"=refnum, "CWDSLib._DCWData"=refnum, "OnDataUpdated"=0, "OnStatusUpdated"=0}}, "AT VentPMACExtended"={"Tag Name"="S060.PXI.Signals.PlltData.SN", "Network Path"="172.15.51.1,1,0", "use opc"=FALSE, "DataSocket Reference"={"CWDSLib._DCWDataSocket"=refnum, "CWDSLib._DCWData"=refnum, "OnDataUpdated"=0, "OnStatusUpdated"=0}}, "Good Frame Barcode"={"Tag Name"="S060.PXI.Signals.PlltData.SN", "Network Path"="172.15.51.1,1,0", "use opc"=FALSE, "DataSocket Reference"={"CWDSLib._DCWDataSocket"=refnum, "CWDSLib._DCWData"=refnum, "OnDataUpdated"=0, "OnStatusUpdated"=0}}, "Bad Frame Barcode"={"Tag Name"="S060.PXI.Signals.PlltData.SN", "Network Path"="172.15.51.1,1,0", "use opc"=FALSE, "DataSocket Reference"={"CWDSLib._DCWDataSocket"=refnum, "CWDSLib._DCWData"=refnum, "OnDataUpdated"=0, "OnStatusUpdated"=0}}, "Extend Z LVDTS"={"Tag Name"="S060.PXI.Signals.PlltData.SN", "Network Path"="172.15.51.1,1,0", "use opc"=FALSE, "DataSocket Reference"={"CWDSLib._DCWDataSocket"=refnum, "CWDSLib._DCWData"=refnum, "OnDataUpdated"=0, "OnStatusUpdated"=0}}, "NVH SunRoof Moving"={"Tag Name"="S060.PXI.Signals.PlltData.SN", "Network Path"="172.15.51.1,1,0", "use opc"=FALSE, "DataSocket Reference"={"CWDSLib._DCWDataSocket"=refnum, "CWDSLib._DCWData"=refnum, "OnDataUpdated"=0, "OnStatusUpdated"=0}}, "NVH SunRoof Stop"={"Tag Name"="S060.PXI.Signals.PlltData.SN", "Network Path"="172.15.51.1,1,0", "use opc"=FALSE, "DataSocket Reference"={"CWDSLib._DCWDataSocket"=refnum, "CWDSLib._DCWData"=refnum, "OnDataUpdated"=0, "OnStatusUpdated"=0}}, "NVH Pass"={"Tag Name"="S060.PXI.Signals.PlltData.SN", "Network Path"="172.15.51.1,1,0", "use opc"=FALSE, "DataSocket Reference"={"CWDSLib._DCWDataSocket"=refnum, "CWDSLib._DCWData"=refnum, "OnDataUpdated"=0, "OnStatusUpdated"=0}}, "NVH Fail"={"Tag Name"="S060.PXI.Signals.PlltData.SN", "Network Path"="172.15.51.1,1,0", "use opc"=FALSE, "DataSocket Reference"={"CWDSLib._DCWDataSocket"=refnum, "CWDSLib._DCWData"=refnum, "OnDataUpdated"=0, "OnStatusUpdated"=0}}, "NVH Operator Express Glass Opened"={"Tag Name"="S060.PXI.Signals.PlltData.SN", "Network Path"="172.15.51.1,1,0", "use opc"=FALSE, "DataSocket Reference"={"CWDSLib._DCWDataSocket"=refnum, "CWDSLib._DCWData"=refnum, "OnDataUpdated"=0, "OnStatusUpdated"=0}}, "NVH Operator Express Glass Closed"={"Tag Name"="S060.PXI.Signals.PlltData.SN", "Network Path"="172.15.51.1,1,0", "use opc"=FALSE, "DataSocket Reference"={"CWDSLib._DCWDataSocket"=refnum, "CWDSLib._DCWData"=refnum, "OnDataUpdated"=0, "OnStatusUpdated"=0}}, "NVH Operator Express Rollo Opened01"={"Tag Name"="S060.PXI.Signals.PlltData.SN", "Network Path"="172.15.51.1,1,0", "use opc"=FALSE, "DataSocket Reference"={"CWDSLib._DCWDataSocket"=refnum, "CWDSLib._DCWData"=refnum, "OnDataUpdated"=0, "OnStatusUpdated"=0}}, "NVH Operator Express Rollo Closed01"={"Tag Name"="S060.PXI.Signals.PlltData.SN", "Network Path"="172.15.51.1,1,0", "use opc"=FALSE, "DataSocket Reference"={"CWDSLib._DCWDataSocket"=refnum, "CWDSLib._DCWData"=refnum, "OnDataUpdated"=0, "OnStatusUpdated"=0}}, "NVH Operator Express Rollo Opened02"={"Tag Name"="S060.PXI.Signals.PlltData.SN", "Network Path"="172.15.51.1,1,0", "use opc"=FALSE, "DataSocket Reference"={"CWDSLib._DCWDataSocket"=refnum, "CWDSLib._DCWData"=refnum, "OnDataUpdated"=0, "OnStatusUpdated"=0}}, "NVH Operator Pass"={"Tag Name"="S060.PXI.Signals.PlltData.SN", "Network Path"="172.15.51.1,1,0", "use opc"=FALSE, "DataSocket Reference"={"CWDSLib._DCWDataSocket"=refnum, "CWDSLib._DCWData"=refnum, "OnDataUpdated"=0, "OnStatusUpdated"=0}}, "NVH Operator Fail"={"Tag Name"="S060.PXI.Signals.PlltData.SN", "Network Path"="172.15.51.1,1,0", "use opc"=FALSE, "DataSocket Reference"={"CWDSLib._DCWDataSocket"=refnum, "CWDSLib._DCWData"=refnum, "OnDataUpdated"=0, "OnStatusUpdated"=0}}, "NVH Operator Check"={"Tag Name"="S060.PXI.Signals.PlltData.SN", "Network Path"="172.15.51.1,1,0", "use opc"=FALSE, "DataSocket Reference"={"CWDSLib._DCWDataSocket"=refnum, "CWDSLib._DCWData"=refnum, "OnDataUpdated"=0, "OnStatusUpdated"=0}}, "NVH Operator Vent Open Noise"={"Tag Name"="S060.PXI.Signals.PlltData.SN", "Network Path"="172.15.51.1,1,0", "use opc"=FALSE, "DataSocket Reference"={"CWDSLib._DCWDataSocket"=refnum, "CWDSLib._DCWData"=refnum, "OnDataUpdated"=0, "OnStatusUpdated"=0}}, "NVH Operator Vent Close Noise"={"Tag Name"="S060.PXI.Signals.PlltData.SN", "Network Path"="172.15.51.1,1,0", "use opc"=FALSE, "DataSocket Reference"={"CWDSLib._DCWDataSocket"=refnum, "CWDSLib._DCWData"=refnum, "OnDataUpdated"=0, "OnStatusUpdated"=0}}, "NVH Operator Sunshade Open Noise"={"Tag Name"="S060.PXI.Signals.PlltData.SN", "Network Path"="172.15.51.1,1,0", "use opc"=FALSE, "DataSocket Reference"={"CWDSLib._DCWDataSocket"=refnum, "CWDSLib._DCWData"=refnum, "OnDataUpdated"=0, "OnStatusUpdated"=0}}, "NVH Operator Sunshade Close Noise"={"Tag Name"="S060.PXI.Signals.PlltData.SN", "Network Path"="172.15.51.1,1,0", "use opc"=FALSE, "DataSocket Reference"={"CWDSLib._DCWDataSocket"=refnum, "CWDSLib._DCWData"=refnum, "OnDataUpdated"=0, "OnStatusUpdated"=0}}, "NVH Operator Glass Open Noise"={"Tag Name"="S060.PXI.Signals.PlltData.SN", "Network Path"="172.15.51.1,1,0", "use opc"=FALSE, "DataSocket Reference"={"CWDSLib._DCWDataSocket"=refnum, "CWDSLib._DCWData"=refnum, "OnDataUpdated"=0, "OnStatusUpdated"=0}}, "NVH Operator Glass Close Noise"={"Tag Name"="S060.PXI.Signals.PlltData.SN", "Network Path"="172.15.51.1,1,0", "use opc"=FALSE, "DataSocket Reference"={"CWDSLib._DCWDataSocket"=refnum, "CWDSLib._DCWData"=refnum, "OnDataUpdated"=0, "OnStatusUpdated"=0}}, "NVH Operator Finish"={"Tag Name"="S060.PXI.Signals.PlltData.SN", "Network Path"="172.15.51.1,1,0", "use opc"=FALSE, "DataSocket Reference"={"CWDSLib._DCWDataSocket"=refnum, "CWDSLib._DCWData"=refnum, "OnDataUpdated"=0, "OnStatusUpdated"=0}}, "Barcode01 OK"={"Tag Name"="S060.PXI.Signals.PlltData.SN", "Network Path"="172.15.51.1,1,0", "use opc"=FALSE, "DataSocket Reference"={"CWDSLib._DCWDataSocket"=refnum, "CWDSLib._DCWData"=refnum, "OnDataUpdated"=0, "OnStatusUpdated"=0}}, "Barcode02 OK"={"Tag Name"="S060.PXI.Signals.PlltData.SN", "Network Path"="172.15.51.1,1,0", "use opc"=FALSE, "DataSocket Reference"={"CWDSLib._DCWDataSocket"=refnum, "CWDSLib._DCWData"=refnum, "OnDataUpdated"=0, "OnStatusUpdated"=0}}, "AT set to Vent ATS Test Pos"={"Tag Name"="S060.PXI.Signals.PlltData.SN", "Network Path"="172.15.51.1,1,0", "use opc"=FALSE, "DataSocket Reference"={"CWDSLib._DCWDataSocket"=refnum, "CWDSLib._DCWData"=refnum, "OnDataUpdated"=0, "OnStatusUpdated"=0}}, "AT set to Vent ATS Home Pos"={"Tag Name"="S060.PXI.Signals.PlltData.SN", "Network Path"="172.15.51.1,1,0", "use opc"=FALSE, "DataSocket Reference"={"CWDSLib._DCWDataSocket"=refnum, "CWDSLib._DCWData"=refnum, "OnDataUpdated"=0, "OnStatusUpdated"=0}}, "Move LVDT Adjust Station"={"Tag Name"="S060.PXI.Signals.PlltData.SN", "Network Path"="172.15.51.1,1,0", "use opc"=FALSE, "DataSocket Reference"={"CWDSLib._DCWDataSocket"=refnum, "CWDSLib._DCWData"=refnum, "OnDataUpdated"=0, "OnStatusUpdated"=0}}}, "PLC string read Tags"={"Serial Number"={"Tag Name"="S060.PXI.Signals.PlltData.SN", "Network Path"="172.15.51.1,1,0", "use opc"=FALSE, "DataSocket Reference"={"CWDSLib._DCWDataSocket"=refnum, "CWDSLib._DCWData"=refnum, "OnDataUpdated"=0, "OnStatusUpdated"=0}}, "Pallet Number"={"Tag Name"="S060.PXI.Signals.PlltData.SN", "Network Path"="172.15.51.1,1,0", "use opc"=FALSE, "DataSocket Reference"={"CWDSLib._DCWDataSocket"=refnum, "CWDSLib._DCWData"=refnum, "OnDataUpdated"=0, "OnStatusUpdated"=0}}, "Inalfa Part Number"={"Tag Name"="S060.PXI.Signals.PlltData.SN", "Network Path"="172.15.51.1,1,0", "use opc"=FALSE, "DataSocket Reference"={"CWDSLib._DCWDataSocket"=refnum, "CWDSLib._DCWData"=refnum, "OnDataUpdated"=0, "OnStatusUpdated"=0}}, "Shade Color"={"Tag Name"="S060.PXI.Signals.PlltData.SN", "Network Path"="172.15.51.1,1,0", "use opc"=FALSE, "DataSocket Reference"={"CWDSLib._DCWDataSocket"=refnum, "CWDSLib._DCWData"=refnum, "OnDataUpdated"=0, "OnStatusUpdated"=0}}, "Model Type"={"Tag Name"="S060.PXI.Signals.PlltData.SN", "Network Path"="172.15.51.1,1,0", "use opc"=FALSE, "DataSocket Reference"={"CWDSLib._DCWDataSocket"=refnum, "CWDSLib._DCWData"=refnum, "OnDataUpdated"=0, "OnStatusUpdated"=0}}, "Customer Number"={"Tag Name"="S060.PXI.Signals.PlltData.SN", "Network Path"="172.15.51.1,1,0", "use opc"=FALSE, "DataSocket Reference"={"CWDSLib._DCWDataSocket"=refnum, "CWDSLib._DCWData"=refnum, "OnDataUpdated"=0, "OnStatusUpdated"=0}}, "Part History Number"={"Tag Name"="S060.PXI.Signals.PlltData.SN", "Network Path"="172.15.51.1,1,0", "use opc"=FALSE, "DataSocket Reference"={"CWDSLib._DCWDataSocket"=refnum, "CWDSLib._DCWData"=refnum, "OnDataUpdated"=0, "OnStatusUpdated"=0}}, "Shade 1 Barcode"={"Tag Name"="S060.PXI.Signals.PlltData.SN", "Network Path"="172.15.51.1,1,0", "use opc"=FALSE, "DataSocket Reference"={"CWDSLib._DCWDataSocket"=refnum, "CWDSLib._DCWData"=refnum, "OnDataUpdated"=0, "OnStatusUpdated"=0}}, "Shade 2 Barcode"={"Tag Name"="S060.PXI.Signals.PlltData.SN", "Network Path"="172.15.51.1,1,0", "use opc"=FALSE, "DataSocket Reference"={"CWDSLib._DCWDataSocket"=refnum, "CWDSLib._DCWData"=refnum, "OnDataUpdated"=0, "OnStatusUpdated"=0}}, "Manual Serial Number"={"Tag Name"="S060.PXI.Signals.PlltData.SN", "Network Path"="172.15.51.1,1,0", "use opc"=FALSE, "DataSocket Reference"={"CWDSLib._DCWDataSocket"=refnum, "CWDSLib._DCWData"=refnum, "OnDataUpdated"=0, "OnStatusUpdated"=0}}, "Manual Inalfa Part Number"={"Tag Name"="S060.PXI.Signals.PlltData.SN", "Network Path"="172.15.51.1,1,0", "use opc"=FALSE, "DataSocket Reference"={"CWDSLib._DCWDataSocket"=refnum, "CWDSLib._DCWData"=refnum, "OnDataUpdated"=0, "OnStatusUpdated"=0}}, "Manual Shade Color"={"Tag Name"="S060.PXI.Signals.PlltData.SN", "Network Path"="172.15.51.1,1,0", "use opc"=FALSE, "DataSocket Reference"={"CWDSLib._DCWDataSocket"=refnum, "CWDSLib._DCWData"=refnum, "OnDataUpdated"=0, "OnStatusUpdated"=0}}, "Manual Model Type"={"Tag Name"="S060.PXI.Signals.PlltData.SN", "Network Path"="172.15.51.1,1,0", "use opc"=FALSE, "DataSocket Reference"={"CWDSLib._DCWDataSocket"=refnum, "CWDSLib._DCWData"=refnum, "OnDataUpdated"=0, "OnStatusUpdated"=0}}, "Manual Customer Number"={"Tag Name"="S060.PXI.Signals.PlltData.SN", "Network Path"="172.15.51.1,1,0", "use opc"=FALSE, "DataSocket Reference"={"CWDSLib._DCWDataSocket"=refnum, "CWDSLib._DCWData"=refnum, "OnDataUpdated"=0, "OnStatusUpdated"=0}}, "Manual Part History Number"={"Tag Name"="S060.PXI.Signals.PlltData.SN", "Network Path"="172.15.51.1,1,0", "use opc"=FALSE, "DataSocket Reference"={"CWDSLib._DCWDataSocket"=refnum, "CWDSLib._DCWData"=refnum, "OnDataUpdated"=0, "OnStatusUpdated"=0}}}, "PLC string write Tags"={"barcode station error"={"Tag Name"="S060.PXI.Signals.PlltData.SN", "Network Path"="172.15.51.1,1,0", "use opc"=FALSE, "DataSocket Reference"={"CWDSLib._DCWDataSocket"=refnum, "CWDSLib._DCWData"=refnum, "OnDataUpdated"=0, "OnStatusUpdated"=0}}, "error message 0"={"Tag Name"="S060.PXI.Signals.PlltData.SN", "Network Path"="172.15.51.1,1,0", "use opc"=FALSE, "DataSocket Reference"={"CWDSLib._DCWDataSocket"=refnum, "CWDSLib._DCWData"=refnum, "OnDataUpdated"=0, "OnStatusUpdated"=0}}, "error message 1"={"Tag Name"="S060.PXI.Signals.PlltData.SN", "Network Path"="172.15.51.1,1,0", "use opc"=FALSE, "DataSocket Reference"={"CWDSLib._DCWDataSocket"=refnum, "CWDSLib._DCWData"=refnum, "OnDataUpdated"=0, "OnStatusUpdated"=0}}, "error message 2"={"Tag Name"="S060.PXI.Signals.PlltData.SN", "Network Path"="172.15.51.1,1,0", "use opc"=FALSE, "DataSocket Reference"={"CWDSLib._DCWDataSocket"=refnum, "CWDSLib._DCWData"=refnum, "OnDataUpdated"=0, "OnStatusUpdated"=0}}, "error message 3"={"Tag Name"="S060.PXI.Signals.PlltData.SN", "Network Path"="172.15.51.1,1,0", "use opc"=FALSE, "DataSocket Reference"={"CWDSLib._DCWDataSocket"=refnum, "CWDSLib._DCWData"=refnum, "OnDataUpdated"=0, "OnStatusUpdated"=0}}}, "use opc"=FALSE, "PLC/OPC Path"=""} ("PLC Comms"), error in="错误输入") -> (found=→"ok?":bool, value=→"PLC Comms":T1, error out=→"错误输出":errorcluster)  [unwired: 1 out]
